vi "数据编码.vi"(0 "table输入":string(combo), 1 "仪器参数上传时间":enum16{"精确到小时", "原始时间"}(ring), 5 "错误常量 2":errorcluster caption="错误输入", 7 "仪器参数":string[](array[string]), 9 "QN":string, 11 "参数":string, 13 "MN":string, 14 "PW":string) -> (4 "错误常量":errorcluster caption="错误输出", 15 "通讯包字符串":string)   [LabVIEW 2016, in "数据传输系统-02.lvlib"]
panel:
  out "核查数据发送次数":i32
  out "小时数据发送次数":i32
  out "长度":i32
  in  "数据块":T1
  out "通讯包":T2={"包头（2）"="##", "数据段长度（4）"="", "数据段"="", "CRC校验"="", "包尾"=""}
  # "范例代码：\n\n##0101QN=20160801085857223;ST=32;CN=1062;PW=100000;MN=010000A8900016F000169DC0;Flag=5\n;CP=&&RtdInterval=30&&1C80\\r\\n"
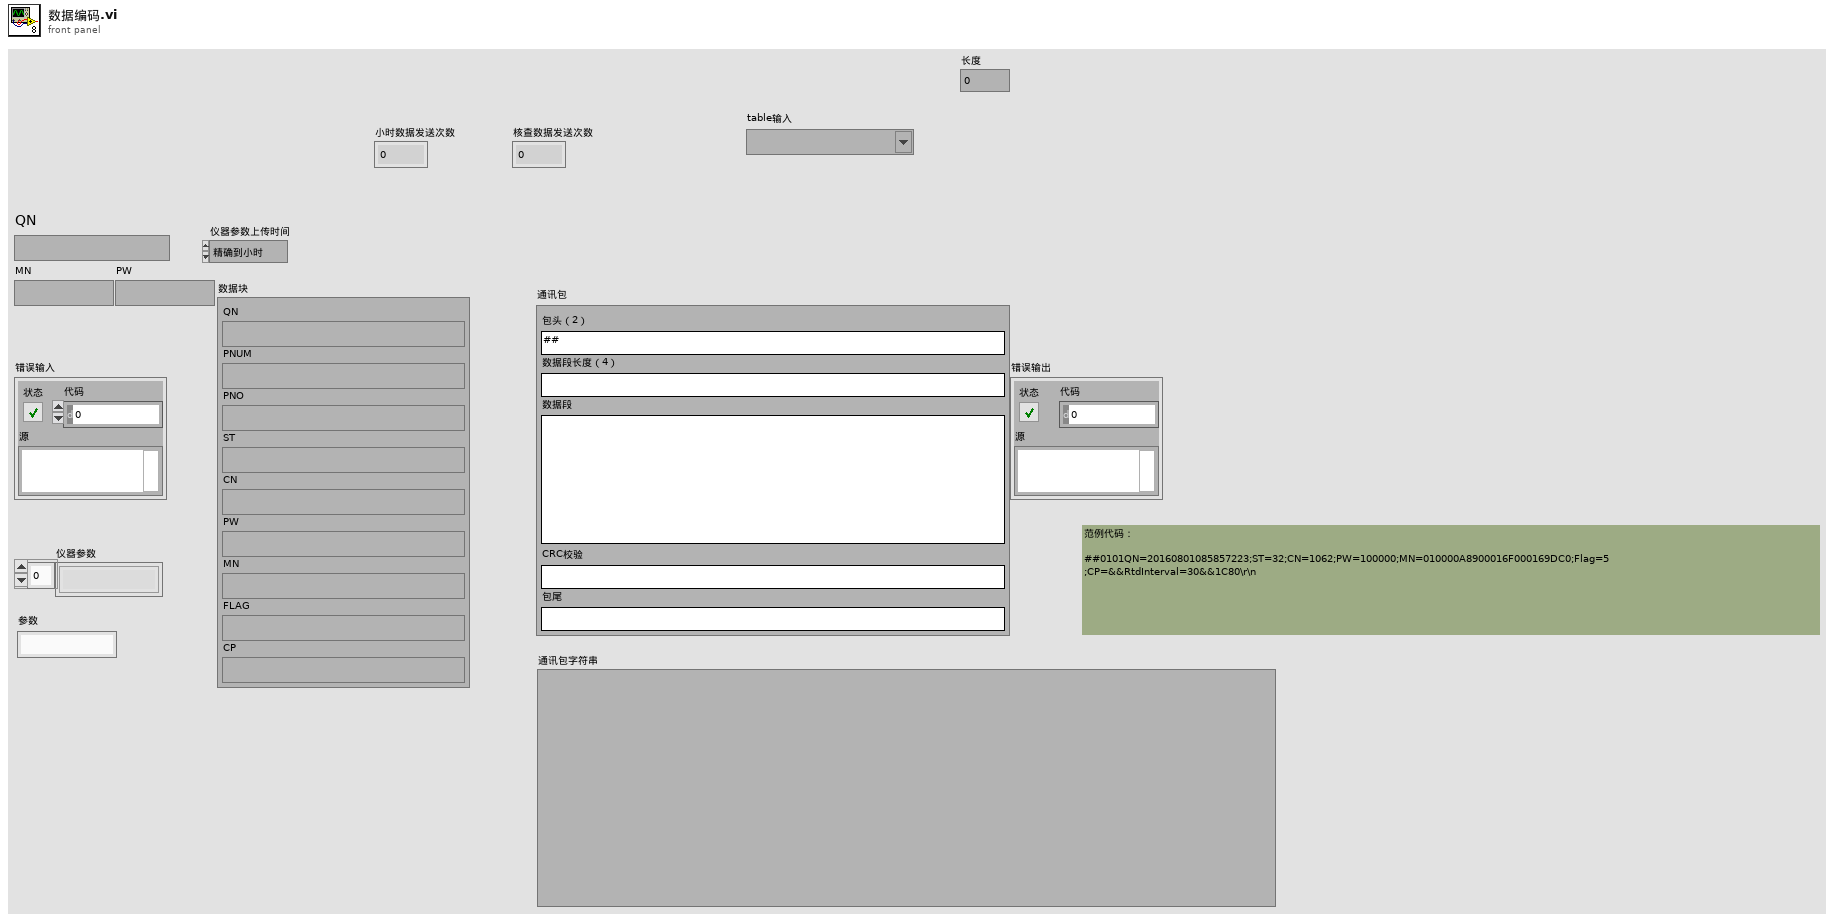
[diagram p1: front panel]
types:
  T1 = cluster{"QN":string, "ST":string, "CN":string, "PW":string, "MN":string, "FLAG":string, "PNUM":string, "PNO":string, "CP":string}
  T2 = cluster{"包头（2）":string, "数据段长度（4）":string, "数据段":string, "CRC校验":string, "包尾":string}
  T3 = cluster{"PH":string[][], "CODCr":string[][], "氨氮":string[][], "CODMn":string[][], "总氮":string[][], "总磷":string[][], "电导率":string[][], "水温":string[][], "DO":string[][], "浊度":string[][], "叶绿素":string[][], "藻密度":string[][], "铜":string[][], "盐度":string[][], "水位":string[][], "流速":string[][], "瞬时流量":string[][], "累积流量":string[][], "亚硝酸盐":string[][], "硫化物":string[][], "ORP":string[][], "铅":string[][], "镉":string[][], "锌":string[][], "镍":string[][], "锰":string[][], "汞":string[][], "气温":string[][], "气压":string[][], "风速":string[][], "风向":string[][], "盐度 2":string[][], "磷酸盐":string[][], "硝氮":string[][], "氟化物":string[][], "挥发酚":string[][], "氯化物":string[][]}
  T4 = enum16{"小时数据", "实时数据", "平行样测试", "集成干预测试", "加标回收测试", "核查数据", "空白零点跨度数据", "提取小时数据", "提取实时数据"}
  T5 = enum16{"小时数据", "实时数据", "平行样测试", "集成干预测试", "加标回收测试", "核查数据", "空白零点跨度数据", "提取小时数据", "提取实时数据", "操作日志"}
  T6 = enum16{"小时数据", "实时数据", "平行样测试", "集成干预测试", "加标回收测试", "核查数据", "空白零点跨度数据", "提取小时数据", "提取实时数据", "操作日志", "仪器参数", "3090仪器参数", "提取仪器参数", "报警信息"}
  T7 = cluster{"CODMn固件信息":string, "氨氮固件信息":string, "总磷固件信息":string, "总氮固件信息":string, "CODCr固件信息":string}
  T8 = typedef "数据传输系统-02.lvlib/应用环境.ctl" = enum16{"STD", "GB212", "婉仪平台"}
  T9 = cluster{"CODMn":dbl, "CODCr":dbl, "DO":dbl, "铜":dbl, "PH":dbl, "氨氮":dbl, "比电导率":dbl, "水温":dbl, "COD":dbl, "浊度":dbl, "总氮":dbl, "总磷":dbl, "叶绿素a":dbl, "藻密度":dbl, "水位":dbl, "流速":dbl, "瞬时流量":dbl, "累积流量":dbl, "亚硝酸盐":dbl, "硫化物":dbl, "ORP":dbl, "铅":dbl, "镉":dbl, "锌":dbl, "镍":dbl, "锰":dbl, "汞":dbl, "气温":dbl, "气压":dbl, "风速":dbl, "风向":dbl, "盐度":dbl, "磷酸盐":dbl, "硝氮":dbl, "氟化物":dbl, "挥发酚":dbl, "氯化物":dbl}
  T10 = cluster{"CODMn":string, "CODCr":string, "DO":string, "铜":string, "PH":string, "氨氮":string, "比电导率":string, "水温":string, "COD":string, "浊度":string, "总氮":string, "总磷":string, "叶绿素a":string, "藻密度":string, "水位":string, "流速":string, "瞬时流量":string, "累积流量":string, "亚硝酸盐":string, "硫化物":string, "ORP":string, "铅":string, "镉":string, "锌":string, "镍":string, "锰":string, "汞":string, "气温":string, "气压":string, "风速":string, "风向":string, "盐度":string, "磷酸盐":string, "硝氮":string, "氟化物":string, "挥发酚":string, "氯化物":string}
  T11 = typedef "LVDateTimeRec.ctl" = cluster{"秒数的小数部分":dbl, "秒":i32, "分":i32, "时":i32, "日":i32, "月":i32, "年":i32, "天数（周）":i32, "天数（年）":i32, "DST":i32}
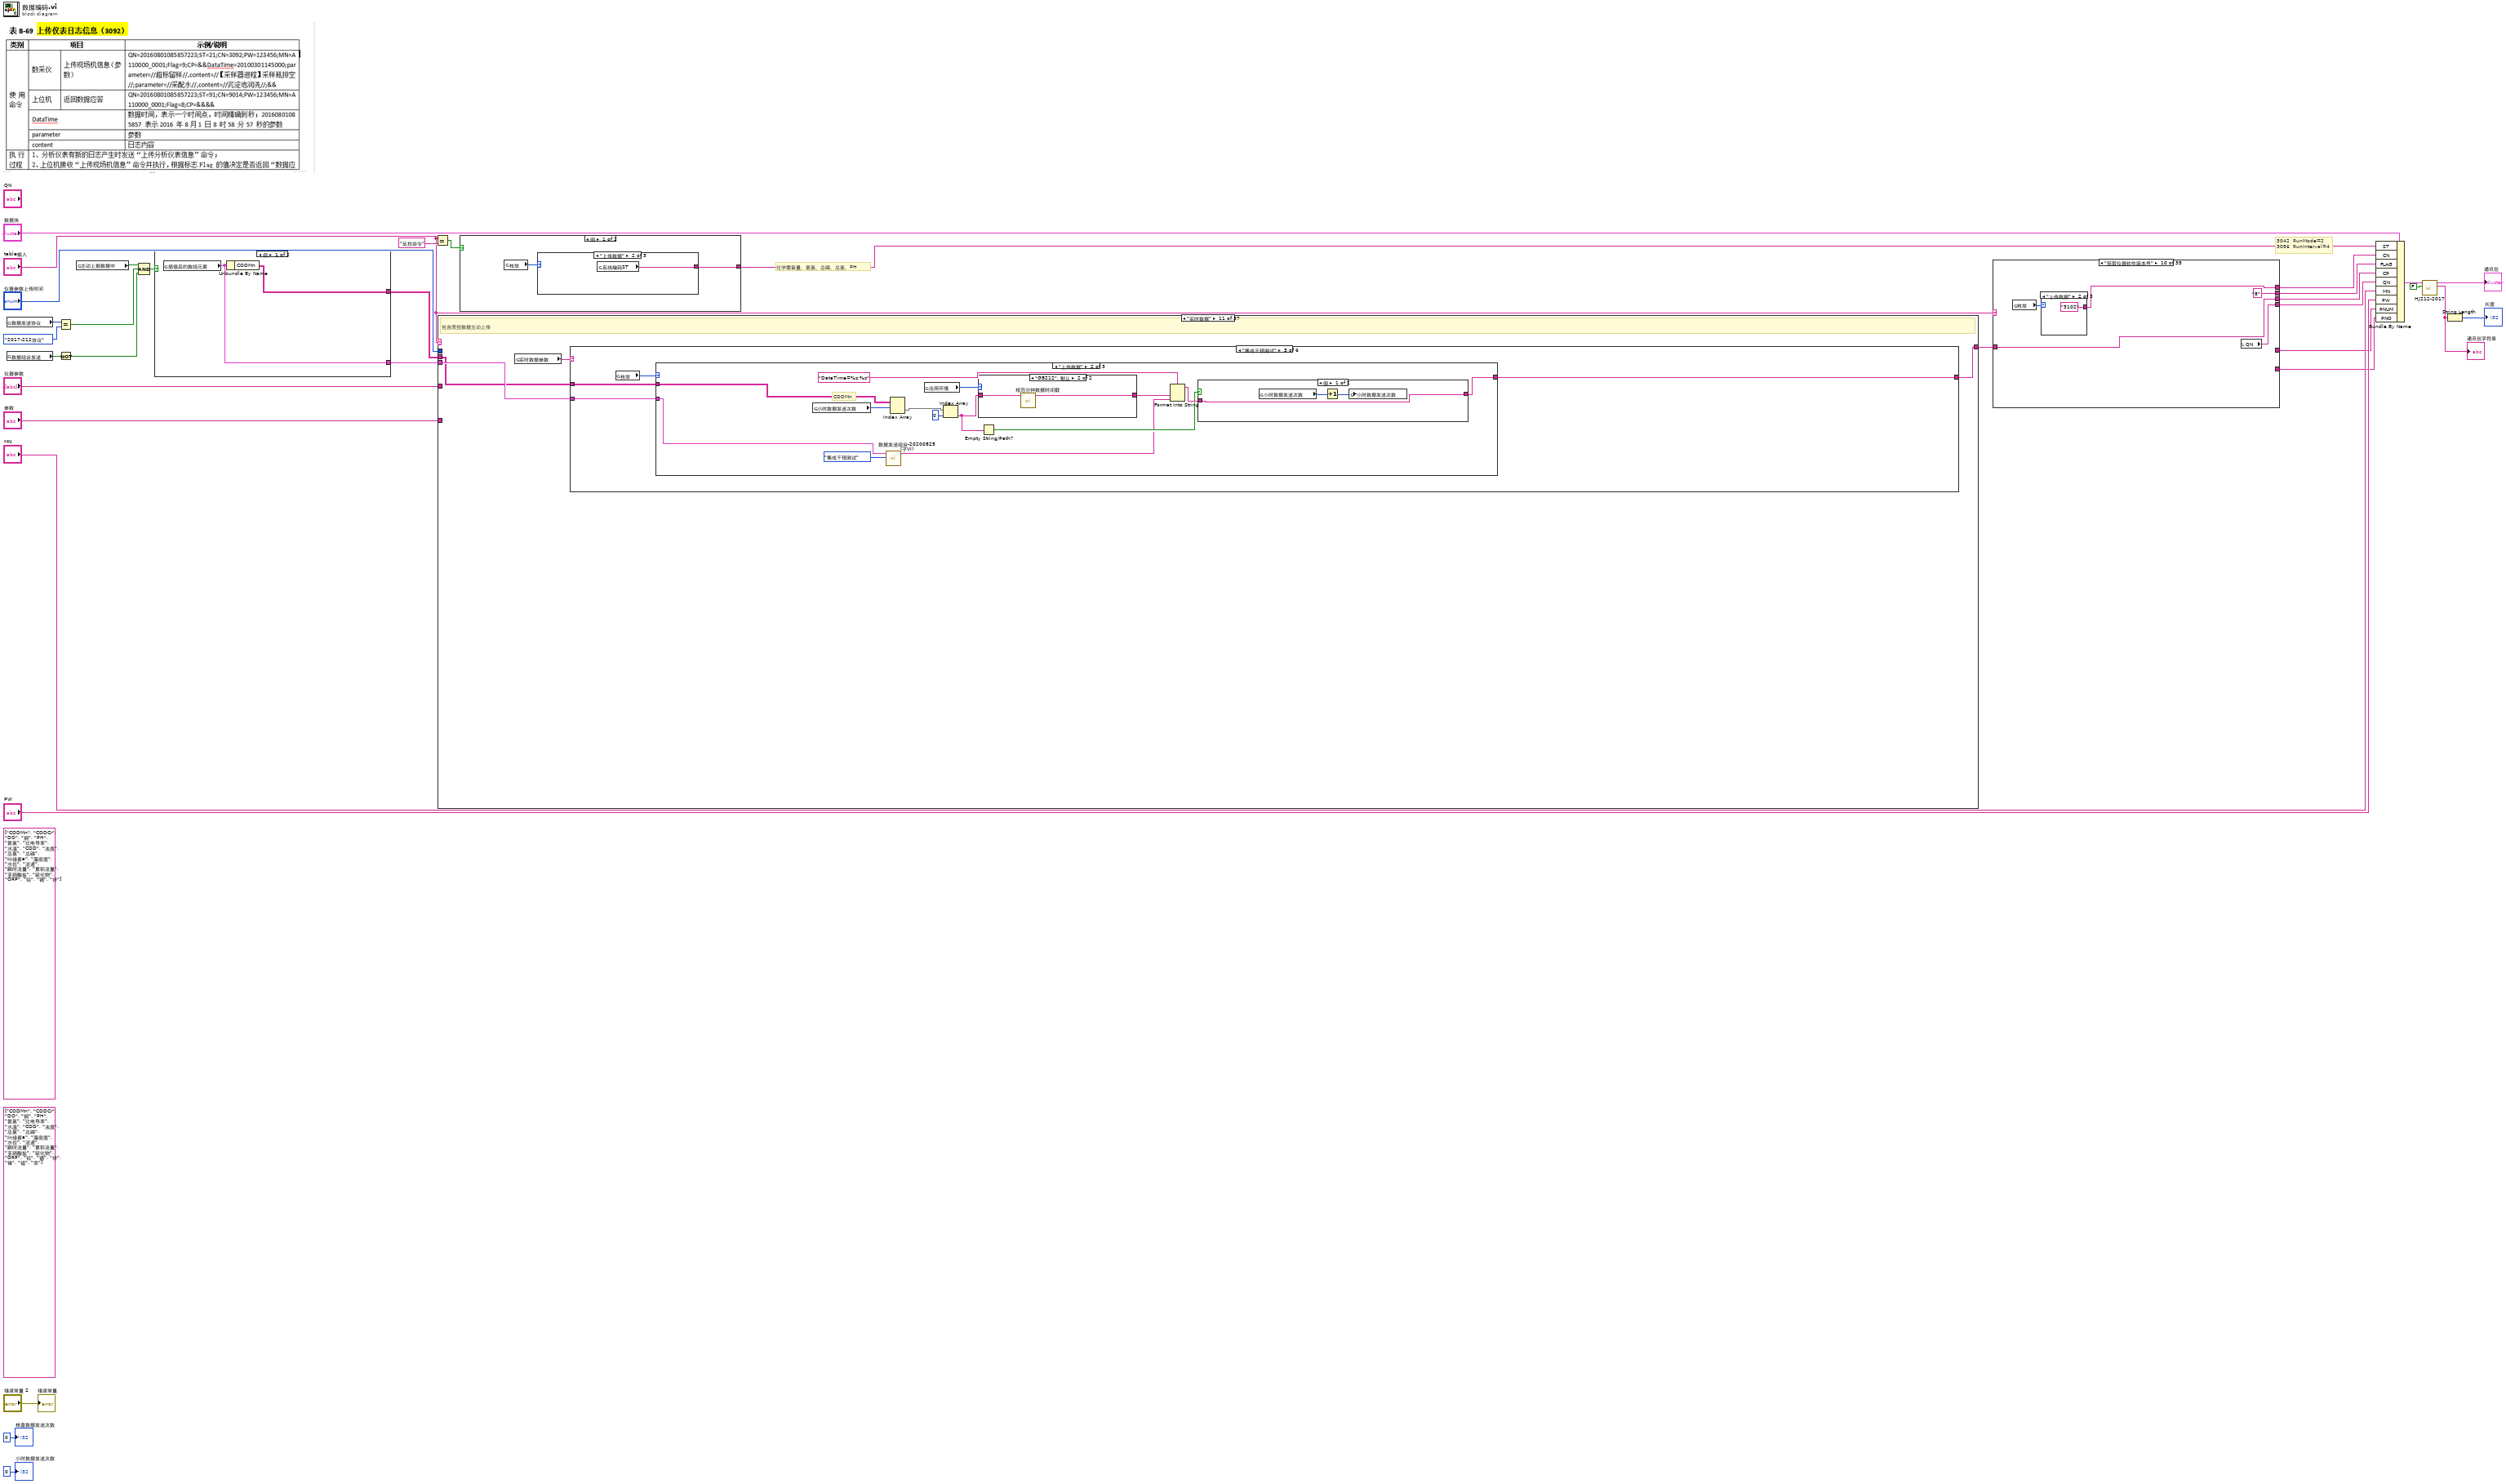
[diagram p0: block diagram]
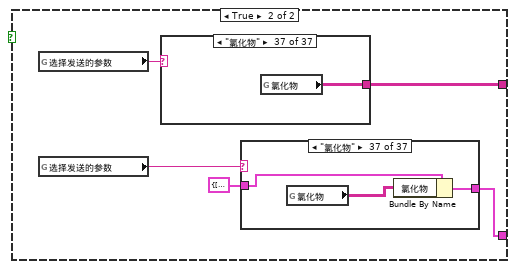
[diagram p2: hidden frame]
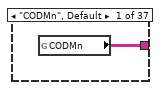
[diagram p3: hidden frame]
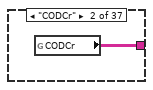
[diagram p4: hidden frame]
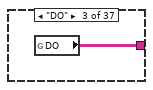
[diagram p5: hidden frame]
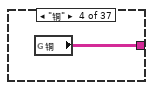
[diagram p6: hidden frame]
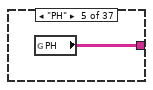
[diagram p7: hidden frame]
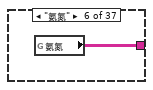
[diagram p8: hidden frame]
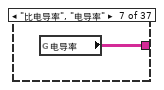
[diagram p9: hidden frame]
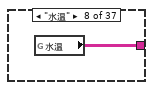
[diagram p10: hidden frame]
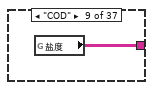
[diagram p11: hidden frame]
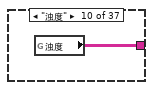
[diagram p12: hidden frame]
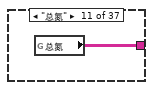
[diagram p13: hidden frame]
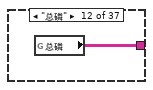
[diagram p14: hidden frame]
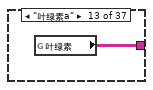
[diagram p15: hidden frame]
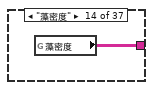
[diagram p16: hidden frame]
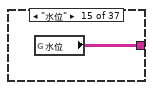
[diagram p17: hidden frame]
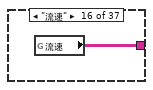
[diagram p18: hidden frame]
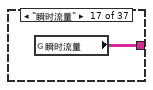
[diagram p19: hidden frame]
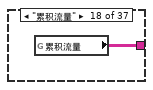
[diagram p20: hidden frame]
diagram:
  (unwired) string[] ["CODMn", "CODCr", "DO", "铜", "PH", "氨氮", "比电导率", "水温", "COD", "浊度", "总氮", "总磷", "叶绿素a", "藻密度", "水位", "流速", "瞬时流量", "累积流量", "亚硝酸盐", "硫化物", "ORP", "铅", "镉", "锌"] ("数组")
  (unwired) string[] ["CODMn", "CODCr", "DO", "铜", "PH", "氨氮", "比电导率", "水温", "COD", "浊度", "总氮", "总磷", "叶绿素a", "藻密度", "水位", "流速", "瞬时流量", "累积流量", "亚硝酸盐", "硫化物", "ORP", "铅", "镉", "锌", "镍", "锰", "汞"] ("数组")
  # "化学需氧量、氨氮、总磷、总氮、PH"
  # "3042  RunMode=2\n3056  RunInterval=4"
  n1 = global read "断电保存全局.vi" "数据发送协议"() -> (w11:enum16{"2005-212协议", "2017-212协议"})
  n2 = global read "断电保存全局.vi" "数据组合发送"() -> (w13:bool)
  n3 = Equal?(x=w11, y=enum16{"2005-212协议", "2017-212协议"}."2017-212协议" ("数据发送版本")) -> (x = y?=w14:bool)
  n4 = Not(x=w13) -> (.not. x?=w12:bool)
  n5 = global read "全局 数据发送重叠.vi" "主动上报数据中"() -> (w18:bool)
  n6 = Compound Arithmetic op=AND ("复合运算")(w18, w14, w12) -> (w15:bool)
  n7 = case shown="假" w15 {
    tunnel: [w36 w40] -> w9
    tunnel: [w35 w38] -> w7
    frame False {
      n8 = global read "插值后的新数组.vi" "插值后的数组元素"() -> (w36:T3)
      n9 = Unbundle By Name(w36) -> ("CODMn"=w35:string[][])
    }
    frame True {
      n10 = global read "全局 水样时间.vi" "选择发送的参数"() -> (w39:string)
      n11 = global read "全局 水样时间.vi" "选择发送的参数"() -> (w41:string)
      n12 = case shown="\"氯化物\"" w39 {
        tunnel: [w42 w43 w44 w45 w46 w47 w48 w49 w50 w51 w52 w53 w54 w55 w56 w57 w58 w59 w60 w61 w62 w63 w64 w65 w66 w67 w68 w69 w70 w71 w72 w73 w74 w75 w76 w77 w78] -> w38
        frame "CODMn", Default {
          n13 = global read "全局 所有参数.vi" "CODMn"() -> (w42:string[][])
        }
        frame "CODCr" {
          n14 = global read "全局 所有参数.vi" "CODCr"() -> (w43:string[][])
        }
        frame "DO" {
          n15 = global read "全局 所有参数.vi" "DO"() -> (w44:string[][])
        }
        frame "铜" {
          n16 = global read "全局 所有参数.vi" "铜"() -> (w45:string[][])
        }
        frame "PH" {
          n17 = global read "全局 所有参数.vi" "PH"() -> (w46:string[][])
        }
        frame "氨氮" {
          n18 = global read "全局 所有参数.vi" "氨氮"() -> (w47:string[][])
        }
        frame "比电导率", "电导率" {
          n19 = global read "全局 所有参数.vi" "电导率"() -> (w48:string[][])
        }
        frame "水温" {
          n20 = global read "全局 所有参数.vi" "水温"() -> (w49:string[][])
        }
        frame "COD" {
          n21 = global read "全局 所有参数.vi" "盐度"() -> (w50:string[][])
        }
        frame "浊度" {
          n22 = global read "全局 所有参数.vi" "浊度"() -> (w51:string[][])
        }
        frame "总氮" {
          n23 = global read "全局 所有参数.vi" "总氮"() -> (w52:string[][])
        }
        frame "总磷" {
          n24 = global read "全局 所有参数.vi" "总磷"() -> (w53:string[][])
        }
        frame "叶绿素a" {
          n25 = global read "全局 所有参数.vi" "叶绿素"() -> (w54:string[][])
        }
        frame "藻密度" {
          n26 = global read "全局 所有参数.vi" "藻密度"() -> (w55:string[][])
        }
        frame "水位" {
          n27 = global read "全局 所有参数.vi" "水位"() -> (w56:string[][])
        }
        frame "流速" {
          n28 = global read "全局 所有参数.vi" "流速"() -> (w57:string[][])
        }
        frame "瞬时流量" {
          n29 = global read "全局 所有参数.vi" "瞬时流量"() -> (w58:string[][])
        }
        frame "累积流量" {
          n30 = global read "全局 所有参数.vi" "累积流量"() -> (w59:string[][])
        }
        frame "亚硝氮" {
          n31 = global read "全局 所有参数.vi" "亚硝酸盐"() -> (w60:string[][])
        }
        frame "硫化物" {
          n32 = global read "全局 所有参数.vi" "硫化物"() -> (w61:string[][])
        }
        frame "ORP" {
          n33 = global read "全局 所有参数.vi" "ORP"() -> (w62:string[][])
        }
        frame "铅" {
          n34 = global read "全局 所有参数.vi" "铅"() -> (w63:string[][])
        }
        frame "镉" {
          n35 = global read "全局 所有参数.vi" "镉"() -> (w64:string[][])
        }
        frame "锌" {
          n36 = global read "全局 所有参数.vi" "锌"() -> (w65:string[][])
        }
        frame "镍" {
          n37 = global read "全局 所有参数.vi" "镍"() -> (w66:string[][])
        }
        frame "锰" {
          n38 = global read "全局 所有参数.vi" "锰"() -> (w67:string[][])
        }
        frame "汞" {
          n39 = global read "全局 所有参数.vi" "汞"() -> (w68:string[][])
        }
        frame "气温" {
          n40 = global read "全局 所有参数.vi" "气温"() -> (w69:string[][])
        }
        frame "气压" {
          n41 = global read "全局 所有参数.vi" "气压"() -> (w70:string[][])
        }
        frame "风速" {
          n42 = global read "全局 所有参数.vi" "风速"() -> (w71:string[][])
        }
        frame "风向" {
          n43 = global read "全局 所有参数.vi" "风向"() -> (w72:string[][])
        }
        frame "盐度" {
          n44 = global read "全局 所有参数.vi" "盐度 2"() -> (w73:string[][])
        }
        frame "磷酸盐" {
          n45 = global read "全局 所有参数.vi" "磷酸盐"() -> (w74:string[][])
        }
        frame "硝氮" {
          n46 = global read "全局 所有参数.vi" "硝氮"() -> (w75:string[][])
        }
        frame "氟化物" {
          n47 = global read "全局 所有参数.vi" "氟化物"() -> (w76:string[][])
        }
        frame "挥发酚" {
          n48 = global read "全局 所有参数.vi" "挥发酚"() -> (w77:string[][])
        }
        frame "氯化物" {
          n49 = global read "全局 所有参数.vi" "氯化物"() -> (w78:string[][])
        }
      }
      n50 = case shown="\"氯化物\"" w41 {
        tunnel: T3 {"PH"=[], "CODCr"=[], "氨氮"=[], "CODMn"=[], "总氮"=[], "总磷"=[], "电导率"=[], "水温"=[], "DO"=[], "浊度"=[], "叶绿素"=[], "藻密度"=[], "铜"=[], "盐度"=[], "水位"=[], "流速"=[], "瞬时流量"=[], "累积流量"=[], "亚硝酸盐"=[], "硫化物"=[], "ORP"=[], "铅"=[], "镉"=[], "锌"=[], "镍"=[], "锰"=[], "汞"=[], "气温"=[], "气压"=[], "风速"=[], "风向"=[], "盐度 2"=[], "磷酸盐"=[], "硝氮"=[], "氟化物"=[], "挥发酚"=[], "氯化物"=[]} ("插值后的数组元素") -> [w80 w84 w87 w90 w93 w96 w99 w102 w105 w108 w111 w114 w117 w119 w123 w126 w128 w131 w134 w137 w140 w143 w146 w149 w152 w155 w158 w161 w164 w167 w170 w173 w176 w179 w182 w185 w188]
        tunnel: [w79 w82 w85 w88 w91 w94 w98 w101 w103 w106 w109 w112 w115 w118 w121 w124 w127 w130 w133 w136 w139 w142 w145 w148 w151 w154 w157 w160 w163 w166 w169 w172 w175 w178 w181 w184 w187] -> w40
        frame "CODMn", Default {
          n51 = global read "全局 所有参数.vi" "CODMn"() -> (w81:string[][])
          n52 = Bundle By Name(cluster=w80, "CODMn"=w81) -> (w79:T3)
        }
        frame "CODCr" {
          n53 = global read "全局 所有参数.vi" "CODCr"() -> (w83:string[][])
          n54 = Bundle By Name(cluster=w84, "CODCr"=w83) -> (w82:T3)
        }
        frame "DO" {
          n55 = global read "全局 所有参数.vi" "DO"() -> (w86:string[][])
          n56 = Bundle By Name(cluster=w87, "DO"=w86) -> (w85:T3)
        }
        frame "铜" {
          n57 = global read "全局 所有参数.vi" "铜"() -> (w89:string[][])
          n58 = Bundle By Name(cluster=w90, "铜"=w89) -> (w88:T3)
        }
        frame "PH" {
          n59 = global read "全局 所有参数.vi" "PH"() -> (w92:string[][])
          n60 = Bundle By Name(cluster=w93, "PH"=w92) -> (w91:T3)
        }
        frame "氨氮" {
          n61 = global read "全局 所有参数.vi" "氨氮"() -> (w95:string[][])
          n62 = Bundle By Name(cluster=w96, "氨氮"=w95) -> (w94:T3)
        }
        frame "比电导率", "电导率" {
          n63 = global read "全局 所有参数.vi" "电导率"() -> (w97:string[][])
          n64 = Bundle By Name(cluster=w99, "电导率"=w97) -> (w98:T3)
        }
        frame "水温" {
          n65 = global read "全局 所有参数.vi" "水温"() -> (w100:string[][])
          n66 = Bundle By Name(cluster=w102, "水温"=w100) -> (w101:T3)
        }
        frame "COD" {
          n67 = global read "全局 所有参数.vi" "盐度"() -> (w104:string[][])
          n68 = Bundle By Name(cluster=w105, "盐度"=w104) -> (w103:T3)
        }
        frame "浊度" {
          n69 = global read "全局 所有参数.vi" "浊度"() -> (w107:string[][])
          n70 = Bundle By Name(cluster=w108, "浊度"=w107) -> (w106:T3)
        }
        frame "总氮" {
          n71 = global read "全局 所有参数.vi" "总氮"() -> (w110:string[][])
          n72 = Bundle By Name(cluster=w111, "总氮"=w110) -> (w109:T3)
        }
        frame "总磷" {
          n73 = global read "全局 所有参数.vi" "总磷"() -> (w113:string[][])
          n74 = Bundle By Name(cluster=w114, "总磷"=w113) -> (w112:T3)
        }
        frame "叶绿素a" {
          n75 = global read "全局 所有参数.vi" "叶绿素"() -> (w116:string[][])
          n76 = Bundle By Name(cluster=w117, "叶绿素"=w116) -> (w115:T3)
        }
        frame "藻密度" {
          n77 = global read "全局 所有参数.vi" "藻密度"() -> (w120:string[][])
          n78 = Bundle By Name(cluster=w119, "藻密度"=w120) -> (w118:T3)
        }
        frame "水位" {
          n79 = global read "全局 所有参数.vi" "水位"() -> (w122:string[][])
          n80 = Bundle By Name(cluster=w123, "水位"=w122) -> (w121:T3)
        }
        frame "流速" {
          n81 = global read "全局 所有参数.vi" "流速"() -> (w125:string[][])
          n82 = Bundle By Name(cluster=w126, "流速"=w125) -> (w124:T3)
        }
        frame "瞬时流量" {
          n83 = global read "全局 所有参数.vi" "瞬时流量"() -> (w129:string[][])
          n84 = Bundle By Name(cluster=w128, "瞬时流量"=w129) -> (w127:T3)
        }
        frame "累积流量" {
          n85 = global read "全局 所有参数.vi" "累积流量"() -> (w132:string[][])
          n86 = Bundle By Name(cluster=w131, "累积流量"=w132) -> (w130:T3)
        }
        frame "亚硝氮" {
          n87 = global read "全局 所有参数.vi" "亚硝酸盐"() -> (w135:string[][])
          n88 = Bundle By Name(cluster=w134, "亚硝酸盐"=w135) -> (w133:T3)
        }
        frame "硫化物" {
          n89 = global read "全局 所有参数.vi" "硫化物"() -> (w138:string[][])
          n90 = Bundle By Name(cluster=w137, "硫化物"=w138) -> (w136:T3)
        }
        frame "ORP" {
          n91 = global read "全局 所有参数.vi" "ORP"() -> (w141:string[][])
          n92 = Bundle By Name(cluster=w140, "ORP"=w141) -> (w139:T3)
        }
        frame "铅" {
          n93 = global read "全局 所有参数.vi" "铅"() -> (w144:string[][])
          n94 = Bundle By Name(cluster=w143, "铅"=w144) -> (w142:T3)
        }
        frame "镉" {
          n95 = global read "全局 所有参数.vi" "镉"() -> (w147:string[][])
          n96 = Bundle By Name(cluster=w146, "镉"=w147) -> (w145:T3)
        }
        frame "锌" {
          n97 = global read "全局 所有参数.vi" "锌"() -> (w150:string[][])
          n98 = Bundle By Name(cluster=w149, "锌"=w150) -> (w148:T3)
        }
        frame "镍" {
          n99 = global read "全局 所有参数.vi" "镍"() -> (w153:string[][])
          n100 = Bundle By Name(cluster=w152, "镍"=w153) -> (w151:T3)
        }
        frame "锰" {
          n101 = global read "全局 所有参数.vi" "锰"() -> (w156:string[][])
          n102 = Bundle By Name(cluster=w155, "锰"=w156) -> (w154:T3)
        }
        frame "汞" {
          n103 = global read "全局 所有参数.vi" "汞"() -> (w159:string[][])
          n104 = Bundle By Name(cluster=w158, "汞"=w159) -> (w157:T3)
        }
        frame "气温" {
          n105 = global read "全局 所有参数.vi" "气温"() -> (w162:string[][])
          n106 = Bundle By Name(cluster=w161, "气温"=w162) -> (w160:T3)
        }
        frame "气压" {
          n107 = global read "全局 所有参数.vi" "气压"() -> (w165:string[][])
          n108 = Bundle By Name(cluster=w164, "气压"=w165) -> (w163:T3)
        }
        frame "风速" {
          n109 = global read "全局 所有参数.vi" "风速"() -> (w168:string[][])
          n110 = Bundle By Name(cluster=w167, "风速"=w168) -> (w166:T3)
        }
        frame "风向" {
          n111 = global read "全局 所有参数.vi" "风向"() -> (w171:string[][])
          n112 = Bundle By Name(cluster=w170, "风向"=w171) -> (w169:T3)
        }
        frame "盐度" {
          n113 = global read "全局 所有参数.vi" "盐度 2"() -> (w174:string[][])
          n114 = Bundle By Name(cluster=w173, "盐度 2"=w174) -> (w172:T3)
        }
        frame "磷酸盐" {
          n115 = global read "全局 所有参数.vi" "磷酸盐"() -> (w177:string[][])
          n116 = Bundle By Name(cluster=w176, "磷酸盐"=w177) -> (w175:T3)
        }
        frame "硝氮" {
          n117 = global read "全局 所有参数.vi" "硝氮"() -> (w180:string[][])
          n118 = Bundle By Name(cluster=w179, "硝氮"=w180) -> (w178:T3)
        }
        frame "氟化物" {
          n119 = global read "全局 所有参数.vi" "氟化物"() -> (w183:string[][])
          n120 = Bundle By Name(cluster=w182, "氟化物"=w183) -> (w181:T3)
        }
        frame "挥发酚" {
          n121 = global read "全局 所有参数.vi" "挥发酚"() -> (w186:string[][])
          n122 = Bundle By Name(cluster=w185, "挥发酚"=w186) -> (w184:T3)
        }
        frame "氯化物" {
          n123 = global read "全局 所有参数.vi" "氯化物"() -> (w189:string[][])
          n124 = Bundle By Name(cluster=w188, "氯化物"=w189) -> (w187:T3)
        }
      }
    }
  }
  n125 = Equal?(x="table输入", y="反控命令") -> (x = y?=w24:bool)
  n126 = case shown="\"实时数据\"" "table输入" {
    tunnel: [w191 w198 w212 w254 w292 _ w306 w315 w322 w332 w343 w498 w529 w580 w628 w680 w709 w741 w772 w798 w827 w856 w893 w926 w959 w998 w1159 w1201 w1362 w1390 w1413 w1446 w1469 w1480 w1488 w1498 w1508] -> w19
    tunnel: w7 -> [_ _ _ _ _ _ _ _ _ _ w340 w497 _ _ _ w679 w710 w736 w767 w799 w826 w855 w892 _ _ _ _ _ w1361 _ w1412 _ _ _ _ _ _]
    tunnel: w9 -> [_ _ _ _ _ _ _ _ _ _ w341 w499 _ _ _ w675 w705 w737 w768 w797 w825 w854 w888 _ _ _ _ _ w1357 w1388 w1408 _ _ _ _ _ _]
    tunnel: "仪器参数" -> [_ _ _ _ _ _ _ _ _ _ _ _ _ _ _ _ _ _ _ _ _ _ _ _ _ w994 w1157 w1197 _ _ _ _ _ _ _ _ _]
    tunnel: "参数" -> [_ _ _ _ _ _ _ _ _ _ _ _ _ _ _ _ _ _ _ _ _ _ _ _ _ w996 _ w1199 _ _ _ _ _ _ _ _ _]
    tunnel: "仪器参数上传时间" -> [_ _ _ _ _ _ _ _ _ _ _ _ _ _ _ _ _ _ _ _ _ _ _ _ _ w993 w1156 w1196 _ _ _ _ _ _ _ _ _]
    frame "反控命令" {
      n127 = global read "全局 反控命令枚举.vi" "反控命令枚举"() -> (w190:enum16{"返回请求应答", "返回执行结果"})
      n128 = case shown="\"返回执行结果\"" w190 {
        tunnel: ["QnRtn=1" w194] -> w191
        frame "返回请求应答", Default {
        }
        frame "返回执行结果" {
          n129 = global read "全局 反控命令枚举.vi" "执行结果定义"() -> (w195:u16)
          n130 = Number To Decimal String(number=w195) -> (decimal integer string=w193:string)  [unwired: 1 in]
          n131 = Concatenate Strings("ExeRtn=", w193) -> (w194:string)
        }
      }
    }
    frame "超标留样返回" {
      n132 = global read "全局1.vi" "枚举"() -> (w197:enum16{"返回请求应答", "上传数据", "返回执行结果"})
      n133 = case shown="\"返回执行结果\"" w197 {
        tunnel: ["QnRtn=1" w200 "ExeRtn=1"] -> w198
        frame "返回请求应答", Default {
        }
        frame "上传数据" {
          n134 = global read "全局1.vi" "register values"() -> (w209:u16[])
          n135 = Get Date/Time In Seconds() -> (seconds since 1Jan1904=w207:timestamp)
          n136 = Index Array(array=w209, index=7 ("索引")) -> (element=w202:u16)
          n137 = Format Date/Time String(time format string (%c)="%Y%m%d%H%M%S" ("时间格式字符串(%c)"), seconds (now)=w207) -> (date/time string=w205:string)  [unwired: 1 in]
          n138 = Number To Decimal String(number=w202) -> (decimal integer string=w203:string)  [unwired: 1 in]
          n139 = Format Into String(format string="VaseNo=%s" ("格式字符串"), w203) -> (resulting string=w201:string)  [unwired: 2 in, 1 out]
          n140 = Format Into String(format string="DataTime=%s;%s" ("格式字符串"), w205, w201) -> (resulting string=w200:string)  [unwired: 2 in, 1 out]
        }
        frame "返回执行结果" {
        }
      }
    }
    frame "提取经纬度环境信息" {
      # "BDS纬度"
      # "BDS纬度"
      # "GPS纬度"
      # "GPS经度"
      # "湿度"
      # "温度"
      # "电压"
      # "时间"
      n141 = global read "全局1.vi" "枚举"() -> (w213:enum16{"返回请求应答", "上传数据", "返回执行结果"})
      n142 = case shown="\"上传数据\"" w213 {
        tunnel: ["QnRtn=1" w226 "ExeRtn=1"] -> w212
        frame "返回请求应答", Default {
        }
        frame "上传数据" {
          n143 = global read "全局 环境参数.vi" "环境参数"() -> (w216:string[][])
          n144 = global read "全局 环境参数.vi" "columns输出"() -> (w223:string[])
          n145 = Index Array(array=w216, index (row)=0 ("索引 (行)")) -> (element=w219:string[])  [unwired: 1 in]
          n146 = Get Date/Time In Seconds() -> (seconds since 1Jan1904=w228:timestamp)
          n147 = Array Subset(array=w223, index=1 ("索引")) -> (w224:string[])  [unwired: 1 in]
          n148 = for {
            tunnel: w224 -> [w232] mode=indexing
            tunnel: [w231] -> w225 mode=indexing
            n149 = case shown="\"BDS经度\"" w232 {
              tunnel: ["" "Volt=%s;" "Temp=%s;" ("格式字符串") "Hum=%s;" ("格式字符串") "Lng=%s;" "Lat=%s;" "Lng2=%s;" "Lat2=%s;"] -> w231
              frame "假", Default {
              }
              frame "电压" {
              }
              frame "室温" {
              }
              frame "湿度" {
              }
              frame "GPS经度" {
              }
              frame "GPS纬度" {
              }
              frame "BDS经度" {
              }
              frame "BDS纬度" {
              }
            }
          }
          n150 = Format Date/Time String(time format string (%c)="%Y%m%d%H%M%S" ("时间格式字符串(%c)"), seconds (now)=w228) -> (date/time string=w227:string)  [unwired: 1 in]
          n151 = Array Subset(array=w219, index=1 ("索引")) -> (w221:string[])  [unwired: 1 in]
          n152 = for {
            shift-right: [w246] -> w215
            shift-left: "" -> [w245]
            tunnel: w225 -> [w244] mode=indexing
            tunnel: w221 -> [w242] mode=indexing
            n153 = Empty String/Path?(string/path=w242) -> (empty?=w248:bool)
            n154 = Fract/Exp String To Number(string=w242) -> (number=w243:dbl)  [unwired: 3 in, 1 out]
            n155 = Number To Fractional String(number=w243) -> (F-format string=w241:string)  [unwired: 3 in]
            n156 = case shown="假" w248 {
              tunnel: [w251 w252] -> w247
              tunnel: w244 -> [w250 _]
              tunnel: w241 -> [w249 _]
              tunnel: w241 -> [_ w252]
              frame False {
                n157 = Format Into String(format string=w250, w249) -> (resulting string=w251:string)  [unwired: 2 in, 1 out]
              }
              frame True {
              }
            }
            n158 = Concatenate Strings(w245, w247) -> (w246:string)
          }
          n159 = Format Into String(format string="DataTime=%s;%s" ("格式字符串"), w227, w215) -> (resulting string=w226:string)  [unwired: 2 in, 1 out]
        }
        frame "返回执行结果" {
        }
      }
    }
    frame "提取现场系统信息" {
      n160 = global read "全局1.vi" "枚举"() -> (w255:enum16{"返回请求应答", "上传数据", "返回执行结果"})
      n161 = case shown="\"上传数据\"" w255 {
        tunnel: ["QnRtn=1" w289 "ExeRtn=1"] -> w254
        frame "返回请求应答", Default {
        }
        frame "上传数据" {
          n162 = global read "全局1.vi" "register values"() -> (w288:u16[])
          n163 = global read "全局1.vi" "系统信息"() -> (w270:u16[])
          n164 = Get Date/Time In Seconds() -> (seconds since 1Jan1904=w275:timestamp)
          n165 = Format Date/Time String(time format string (%c)="%Y%m%d%H%M%S%u" ("时间格式字符串(%c)"), seconds (now)=w275) -> (date/time string=w278:string)  [unwired: 1 in]
          n166 = Number To Decimal String(number=w270) -> (decimal integer string=w269:string[])  [unwired: 1 in]
          n167 = Index Array(array=w288, index #1=0 ("索引"), index #2=6 ("索引")) -> (element #1=w284:u16, element #2=w272:u16)
          n168 = Number To Decimal String(number=w284) -> (decimal integer string=w286:string)  [unwired: 1 in]
          n169 = Number To Decimal String(number=w272) -> (decimal integer string=w281:string)  [unwired: 1 in]
          n170 = Index Array(array=w269) -> (element #1=w267:string, element #2=w264:string, element #3=w261:string, element #4=w258:string)  [unwired: 4 in]
          n171 = Search and Replace String(input string=w278, search string="." ("搜索字符串")) -> (result string=w274:string)  [unwired: 6 in, 3 out]
          n172 = Format Into String(format string="SystemTask=%s;" ("格式字符串"), w267) -> (resulting string=w266:string)  [unwired: 2 in, 1 out]
          n173 = Format Into String(format string="PumpState=%s;" ("格式字符串"), w264) -> (resulting string=w263:string)  [unwired: 2 in, 1 out]
          n174 = Format Into String(format string="AlgClean=%s;" ("格式字符串"), w261) -> (resulting string=w260:string)  [unwired: 2 in, 1 out]
          n175 = Format Into String(format string="SystemAlarm=0%s;" ("格式字符串"), w258) -> (resulting string=w257:string)  [unwired: 2 in, 1 out]
          n176 = Format Into String(format string="RunMode=%s;" ("格式字符串"), w286) -> (resulting string=w271:string)  [unwired: 2 in, 1 out]
          n177 = Format Into String(format string="RunInterval=%s;" ("格式字符串"), w281) -> (resulting string=w282:string)  [unwired: 2 in, 1 out]
          n178 = Format Into String(format string="SystemTime=%s;" ("格式字符串"), w274) -> (resulting string=w279:string)  [unwired: 2 in, 1 out]
          n179 = Concatenate Strings(w271, w263, w266, w260, w257, w282, w279) -> (w289:string)
        }
        frame "返回执行结果" {
        }
      }
    }
    frame "提取监测仪表时间" {
      n180 = global read "全局1.vi" "枚举"() -> (w291:enum16{"返回请求应答", "上传数据", "返回执行结果"})
      n181 = case shown="\"上传数据\"" w291 {
        tunnel: ["QnRtn=1" w304 "ExeRtn=1"] -> w292
        frame "返回请求应答", Default {
        }
        frame "上传数据" {
          n182 = global read "全局 提取仪器参数.vi" "仪器编码"() -> (w294:string)
          n183 = Format Into String(format string="PolId=%s;" ("格式字符串"), w294) -> (resulting string=w302:string)  [unwired: 2 in, 1 out]
          n184 = Get Date/Time In Seconds() -> (seconds since 1Jan1904=w297:timestamp)
          n185 = Format Date/Time String(time format string (%c)="%Y%m%d%H%M%S%u" ("时间格式字符串(%c)"), seconds (now)=w297) -> (date/time string=w300:string)  [unwired: 1 in]
          n186 = Search and Replace String(input string=w300, search string="." ("搜索字符串")) -> (result string=w296:string)  [unwired: 6 in, 3 out]
          n187 = Format Into String(format string="SystemTime=%s;" ("格式字符串"), w296) -> (resulting string=w295:string)  [unwired: 2 in, 1 out]
          n188 = Concatenate Strings(w302, w295) -> (w304:string)
        }
        frame "返回执行结果" {
        }
      }
    }
    frame "心跳包", Default {
    }
    frame "提取数采仪时间" {
      (unwired) ""
      n189 = global read "全局1.vi" "枚举"() -> (w307:enum16{"返回请求应答", "上传数据", "返回执行结果"})
      n190 = case shown="\"上传数据\"" w307 {
        tunnel: ["QnRtn=1" w309 "ExeRtn=1"] -> w306
        frame "返回请求应答", Default {
        }
        frame "上传数据" {
          n191 = Get Date/Time In Seconds() -> (seconds since 1Jan1904=w313:timestamp)
          n192 = Format Date/Time String(time format string (%c)="%Y%m%d%H%M%S" ("时间格式字符串(%c)"), seconds (now)=w313) -> (date/time string=w310:string)  [unwired: 1 in]
          n193 = Concatenate Strings("SystemTime=", w310) -> (w309:string)
        }
        frame "返回执行结果" {
        }
      }
    }
    frame "获取软件版本号" {
      (unwired) ""
      n194 = global read "全局1.vi" "枚举"() -> (w316:enum16{"返回请求应答", "上传数据", "返回执行结果"})
      n195 = case shown="\"上传数据\"" w316 {
        tunnel: ["QnRtn=1" w319 "ExeRtn=1"] -> w315
        frame "返回请求应答", Default {
        }
        frame "上传数据" {
          n196 = global read "全局1.vi" "版本信息"() -> (w318:string)
          n197 = Concatenate Strings("Version=", w318) -> (w319:string)
        }
        frame "返回执行结果" {
        }
      }
    }
    frame "获取仪器软件版本号" {
      (unwired) ""
      n198 = global read "全局1.vi" "枚举"() -> (w323:enum16{"返回请求应答", "上传数据", "返回执行结果"})
      n199 = case shown="\"上传数据\"" w323 {
        tunnel: ["QnRtn=1" w329 "ExeRtn=1"] -> w322
        frame "返回请求应答", Default {
        }
        frame "上传数据" {
          n200 = global read "全局1.vi" "固件版本"() -> (w328:T7)
          n201 = global read "全局 小时数据发送次数.vi" "小时数据发送次数"() -> (w326:i32)
          n202 = Cluster To Array(cluster=w328) -> (array=w327:string[])
          n203 = Index Array(array=w327, index=w326) -> (element=w325:string)
          n204 = Concatenate Strings("FirmwareVersion=", w325) -> (w329:string)
        }
        frame "返回执行结果" {
        }
      }
    }
    frame "提取实时数据间隔" {
      (unwired) ""
      n205 = global read "全局1.vi" "枚举"() -> (w333:enum16{"返回请求应答", "上传数据", "返回执行结果"})
      n206 = case shown="\"上传数据\"" w333 {
        tunnel: ["QnRtn=1" w337 "ExeRtn=1"] -> w332
        frame "返回请求应答", Default {
        }
        frame "上传数据" {
          n207 = global read "实时数据发送间隔全局.vi" "实时数据发送间隔"() -> (w336:u32)
          n208 = Number To Decimal String(number=w336) -> (decimal integer string=w335:string)  [unwired: 1 in]
          n209 = Concatenate Strings("RtdInterval=", w335) -> (w337:string)
        }
        frame "返回执行结果" {
        }
      }
    }
    frame "实时数据" {
      # "包含质控数据主动上传"
      n210 = global read "全局 实时数据参数.vi" "实时数据参数"() -> (w342:string)
      n211 = case shown="\"集成干预测试\"" w342 {
        tunnel: [w346 w371 w396 w427 w451 w472] -> w343
        tunnel: w341 -> [w345 w370 w395 w425 w449 w470]
        tunnel: w340 -> [w344 w369 w394 w424 w448 w469]
        frame "水样测试", Default {
          n212 = global read "全局1.vi" "枚举"() -> (w347:enum16{"返回请求应答", "上传数据", "返回执行结果"})
          n213 = case shown="\"上传数据\"" w347 {
            tunnel: ["QnRtn=1" w365 "ExeRtn=1"] -> w346
            tunnel: w345 -> [_ w351 _]
            tunnel: w344 -> [_ w349 _]
            frame "返回请求应答", Default {
            }
            frame "上传数据" {
              n214 = call "数据发送组合-20200825 (子VI).vi"("枚举"=T4."实时数据", "插值后的数组元素"=w351) -> ("字符串"=w352:string)  [unwired: 9 in]
              n215 = global read "全局 小时数据发送次数.vi" "小时数据发送次数"() -> (w363:i32)
              n216 = Index Array(array=w349, index (row)=w363) -> (element=w362:string[])  [unwired: 1 in]
              n217 = Index Array(array=w362, index=0 ("索引")) -> (element=w360:string)
              n218 = call "规范时间戳.vi"("字符串"=w360) -> ("result string"=w358:string)  [unwired: 10 in]
              n219 = Empty String/Path?(string/path=w352) -> (empty?=w364:bool)
              n220 = Format Into String(format string="DataTime=%s;", w358) -> (resulting string=w357:string)  [unwired: 2 in, 1 out]
              n221 = Concatenate Strings(w357, w352) -> (w354:string)
              n222 = String Length(string=w354) -> (length=w356:i32)
              n223 = Decrement(x=w356) -> (x-1=w355:i32)
              n224 = String Subset(string=w354, length (rest)=w355) -> (substring=w353:string)  [unwired: 1 in]
              n225 = case shown="假" w364 {
                tunnel: [w366 ""] -> w365
                tunnel: w353 -> [w366 _]
                frame False {
                }
                frame True {
                }
              }
            }
            frame "返回执行结果" {
            }
          }
        }
        frame "平行样测试" {
          n226 = global read "全局1.vi" "枚举"() -> (w372:enum16{"返回请求应答", "上传数据", "返回执行结果"})
          n227 = case shown="\"上传数据\"" w372 {
            tunnel: ["QnRtn=1" w384 "ExeRtn=1"] -> w371
            tunnel: w369 -> [_ w378 _]
            tunnel: w370 -> [_ w375 _]
            frame "返回请求应答", Default {
            }
            frame "上传数据" {
              # "CODMn"
              n228 = call "数据发送组合-20200825 (子VI).vi"("枚举"=T4."平行样测试", "插值后的数组元素"=w375) -> ("字符串"=w374:string)  [unwired: 9 in]
              n229 = global read "全局 小时数据发送次数.vi" "小时数据发送次数"() -> (w377:i32)
              n230 = Index Array(array=w378, index (row)=w377) -> (element=w382:string[])  [unwired: 1 in]
              n231 = Index Array(array=w382, index=0 ("索引")) -> (element=w379:string)
              n232 = call "规范时间戳.vi"("字符串"=w379) -> ("result string"=w380:string)  [unwired: 10 in]
              n233 = Empty String/Path?(string/path=w379) -> (empty?=w383:bool)
              n234 = Format Into String(format string="DataTime=%s;%s" ("格式字符串"), w380, w374) -> (resulting string=w385:string)  [unwired: 2 in, 1 out]
              n235 = case shown="真" w383 {
                tunnel: [w389 ""] -> w384
                tunnel: w385 -> [w389 _]
                frame False {
                  n236 = global read "全局 小时数据发送次数.vi" "小时数据发送次数"() -> (w388:i32)
                  n237 = Increment(x=w388) -> (x+1=w387:i32)
                  n238 = global write "全局 小时数据发送次数.vi" "小时数据发送次数"(w387) -> ()
                }
                frame True {
                  n239 = global read "全局 小时数据发送次数.vi" "小时数据发送次数"() -> (w391:i32)
                  n240 = Increment(x=w391) -> (x+1=w390:i32)
                  n241 = global write "全局 小时数据发送次数.vi" "小时数据发送次数"(w390) -> ()
                }
              }
            }
            frame "返回执行结果" {
            }
          }
        }
        frame "集成干预测试" {
          n242 = global read "全局1.vi" "枚举"() -> (w397:enum16{"返回请求应答", "上传数据", "返回执行结果"})
          n243 = case shown="\"上传数据\"" w397 {
            tunnel: ["QnRtn=1" w410 "ExeRtn=1"] -> w396
            tunnel: w394 -> [_ w404 _]
            tunnel: w395 -> [_ w401 _]
            frame "返回请求应答", Default {
            }
            frame "上传数据" {
              # "CODMn"
              n244 = global read "全局 小时数据发送次数.vi" "小时数据发送次数"() -> (w403:i32)
              n245 = call "数据发送组合-20200825 (子VI).vi"("枚举"=T4."集成干预测试", "插值后的数组元素"=w401) -> ("字符串"=w400:string)  [unwired: 9 in]
              n246 = Index Array(array=w404, index (row)=w403) -> (element=w408:string[])  [unwired: 1 in]
              n247 = global read "断电保存全局.vi" "应用环境"() -> (w399:T8)
              n248 = Index Array(array=w408, index=0 ("索引")) -> (element=w405:string)
              n249 = case shown="\"GB212\", 默认" w399 {
                tunnel: [w414 w415] -> w406
                tunnel: w405 -> [w413 w416]
                frame "STD" {
                  n250 = call "规范时间戳.vi"("字符串"=w413) -> ("result string"=w414:string)  [unwired: 10 in]
                }
                frame "GB212", Default {
                  n251 = call "规范分钟数据时间戳.vi"("字符串"=w416) -> ("result string"=w415:string)  [unwired: 10 in]
                }
              }
              n252 = Empty String/Path?(string/path=w405) -> (empty?=w409:bool)
              n253 = Format Into String(format string="DataTime=%s;%s" ("格式字符串"), w406, w400) -> (resulting string=w411:string)  [unwired: 2 in, 1 out]
              n254 = case shown="假" w409 {
                tunnel: [w419 ""] -> w410
                tunnel: w411 -> [w419 _]
                frame False {
                  n255 = global read "全局 小时数据发送次数.vi" "小时数据发送次数"() -> (w418:i32)
                  n256 = Increment(x=w418) -> (x+1=w417:i32)
                  n257 = global write "全局 小时数据发送次数.vi" "小时数据发送次数"(w417) -> ()
                }
                frame True {
                  n258 = global read "全局 小时数据发送次数.vi" "小时数据发送次数"() -> (w421:i32)
                  n259 = Increment(x=w421) -> (x+1=w420:i32)
                  n260 = global write "全局 小时数据发送次数.vi" "小时数据发送次数"(w420) -> ()
                }
              }
            }
            frame "返回执行结果" {
            }
          }
        }
        frame "加标回收测试" {
          n261 = global read "全局1.vi" "枚举"() -> (w426:enum16{"返回请求应答", "上传数据", "返回执行结果"})
          n262 = case shown="\"上传数据\"" w426 {
            tunnel: ["QnRtn=1" w437 "ExeRtn=1"] -> w427
            tunnel: w424 -> [_ w432 _]
            tunnel: w425 -> [_ w434 _]
            frame "返回请求应答", Default {
            }
            frame "上传数据" {
              # "w01001-Check=63.0,w01001-WaterTime=20160801080000,w01001-Water=45.23,w01001-Chroma=1000,w01001-Volume=0.2,w01001-DVolume=200,w01003-Flag=N;"
              # "CODMn"
              n263 = global read "全局 小时数据发送次数.vi" "小时数据发送次数"() -> (w431:i32)
              n264 = call "加标回收数据组合 (子VI).vi"("小时数据发送次数"=w431, "数据"=w432, "污染物编码"="CODMn") -> ("datatime"=w430:string)  [unwired: 7 in, 1 out]
              n265 = call "规范时间戳.vi"("字符串"=w430) -> ("result string"=w439:string)  [unwired: 10 in]
              n266 = Empty String/Path?(string/path=w439) -> (empty?=w436:bool)
              n267 = call "数据发送组合-20200825 (子VI).vi"("枚举"=T4."加标回收测试", "插值后的数组元素"=w434) -> ("字符串"=w433:string)  [unwired: 9 in]
              n268 = Format Into String(format string="DataTime=%s;%s" ("格式字符串"), w439, w433) -> (resulting string=w438:string)  [unwired: 2 in, 1 out]
              n269 = case shown="真" w436 {
                tunnel: [w443 ""] -> w437
                tunnel: w438 -> [w443 _]
                frame False {
                  n270 = global read "全局 小时数据发送次数.vi" "小时数据发送次数"() -> (w442:i32)
                  n271 = Increment(x=w442) -> (x+1=w441:i32)
                  n272 = global write "全局 小时数据发送次数.vi" "小时数据发送次数"(w441) -> ()
                }
                frame True {
                  n273 = global read "全局 小时数据发送次数.vi" "小时数据发送次数"() -> (w445:i32)
                  n274 = Increment(x=w445) -> (x+1=w444:i32)
                  n275 = global write "全局 小时数据发送次数.vi" "小时数据发送次数"(w444) -> ()
                }
              }
            }
            frame "返回执行结果" {
            }
          }
        }
        frame "核查数据" {
          n276 = global read "全局1.vi" "枚举"() -> (w450:enum16{"返回请求应答", "上传数据", "返回执行结果"})
          n277 = case shown="\"上传数据\"" w450 {
            tunnel: ["QnRtn=1" w461 "ExeRtn=1"] -> w451
            tunnel: w449 -> [_ w454 _]
            tunnel: w448 -> [_ w453 _]
            frame "返回请求应答", Default {
            }
            frame "上传数据" {
              # "将非空数组的时间戳写入"
              n278 = global read "全局 小时数据发送次数.vi" "小时数据发送次数"() -> (w457:i32)
              n279 = Index Array(array=w453, index (row)=w457) -> (element=w460:string[])  [unwired: 1 in]
              n280 = call "数据发送组合-20200825 (子VI).vi"("枚举"=T4."核查数据", "插值后的数组元素"=w454) -> ("字符串"=w455:string)  [unwired: 9 in]
              n281 = Index Array(array=w460, index=0 ("索引")) -> (element=w459:string)
              n282 = call "规范分钟数据时间戳.vi"("字符串"=w459) -> ("result string"=w458:string)  [unwired: 10 in]
              n283 = Empty String/Path?(string/path=w458) -> (empty?=w463:bool)
              n284 = Format Into String(format string="DataTime=%s;%s" ("格式字符串"), w458, w455) -> (resulting string=w462:string)  [unwired: 2 in, 1 out]
              n285 = case shown="假" w463 {
                tunnel: [w466 ""] -> w461
                tunnel: w462 -> [w466 _]
                frame False {
                }
                frame True {
                }
              }
            }
            frame "返回执行结果" {
            }
          }
        }
        frame "空白测试", "跨度核查" {
          n286 = global read "全局1.vi" "枚举"() -> (w471:enum16{"返回请求应答", "上传数据", "返回执行结果"})
          n287 = case shown="\"上传数据\"" w471 {
            tunnel: ["QnRtn=1" w483 "ExeRtn=1"] -> w472
            tunnel: w470 -> [_ w479 _]
            tunnel: w469 -> [_ w477 _]
            frame "返回请求应答", Default {
            }
            frame "上传数据" {
              n288 = global read "全局 小时数据发送次数.vi" "小时数据发送次数"() -> (w481:i32)
              n289 = call "数据发送组合-20200825 (子VI).vi"("枚举"=T4."空白零点跨度数据", "插值后的数组元素"=w479) -> ("字符串"=w478:string)  [unwired: 9 in]
              n290 = Index Array(array=w477, index (row)=w481) -> (element=w487:string[])  [unwired: 1 in]
              n291 = Index Array(array=w487, index #1=0 ("索引"), index #2=3 ("索引"), index #3=5 ("索引")) -> (element #1=w475:string, element #3=w476:string)  [unwired: 1 out]
              n292 = case shown="\"pf\"" w476 {
                tunnel: [w490 w492] -> w474
                tunnel: w475 -> [w491 w493]
                frame "假", Default {
                  n293 = call "规范小时时间戳.vi"("字符串"=w491) -> ("result string"=w490:string)  [unwired: 10 in]
                }
                frame "pf" {
                  # "pf数据时间戳不变"
                  n294 = call "规范时间戳.vi"("字符串"=w493) -> ("result string"=w492:string)  [unwired: 10 in]
                }
              }
              n295 = Empty String/Path?(string/path=w474) -> (empty?=w484:bool)
              n296 = Format Into String(format string="DataTime=%s;%s" ("格式字符串"), w474, w478) -> (resulting string=w482:string)  [unwired: 2 in, 1 out]
              n297 = case shown="假" w484 {
                tunnel: [w494 ""] -> w483
                tunnel: w482 -> [w494 _]
                frame False {
                }
                frame True {
                }
              }
            }
            frame "返回执行结果" {
            }
          }
        }
      }
    }
    frame "小时数据" {
      # "发送小时数据"
      n298 = global read "全局1.vi" "枚举"() -> (w500:enum16{"返回请求应答", "上传数据", "返回执行结果"})
      n299 = case shown="\"上传数据\"" w500 {
        tunnel: ["QnRtn=1" w522 "ExeRtn=1"] -> w498
        tunnel: w499 -> [_ w510 _]
        tunnel: w497 -> [_ w507 _]
        frame "返回请求应答", Default {
          (unwired) 0 ("当前包数")
          n300 = global read "全局 数据数组大小.vi" "数据数组大小"() -> (w501:i32)
          n301 = global write "全局1.vi" "枚举"(enum16{"返回请求应答", "上传数据", "返回执行结果"}."上传数据" ("枚举")) -> ()
          n302 = Equal To 0?(x=w501) -> (x = 0?=w502:bool)
          n303 = case shown="真" w502 {
            frame False {
            }
            frame True {
              n304 = global read "全局 小时数据发送次数.vi" "小时数据发送次数"() -> (w506:i32)
              n305 = Increment(x=w506) -> (x+1=w505:i32)
              n306 = global write "全局 小时数据发送次数.vi" "小时数据发送次数"(w505) -> ()
            }
          }
        }
        frame "上传数据" {
          n307 = global read "全局 小时数据发送次数.vi" "小时数据发送次数"() -> (w521:i32)
          n308 = call "数据发送组合-20200825 (子VI).vi"("枚举"=enum16{"小时数据", "实时数据"}."小时数据", "插值后的数组元素"=w510) -> ("字符串"=w508:string)  [unwired: 9 in]
          n309 = Index Array(array=w507, index (row)=w521) -> (element=w520:string[])  [unwired: 1 in]
          n310 = Index Array(array=w520, index=0 ("索引")) -> (element=w518:string)
          n311 = call "规范小时时间戳.vi"("字符串"=w518) -> ("result string"=w515:string)  [unwired: 10 in]
          n312 = Empty String/Path?(string/path=w508) -> (empty?=w523:bool)
          n313 = Format Into String(format string="DataTime=%s;", w515) -> (resulting string=w517:string)  [unwired: 2 in, 1 out]
          n314 = Concatenate Strings(w517, w508) -> (w512:string)
          n315 = String Length(string=w512) -> (length=w514:i32)
          n316 = Decrement(x=w514) -> (x-1=w513:i32)
          n317 = String Subset(string=w512, length (rest)=w513) -> (substring=w511:string)  [unwired: 1 in]
          n318 = case shown="假" w523 {
            tunnel: [w524 ""] -> w522
            tunnel: w511 -> [w524 _]
            frame False {
            }
            frame True {
            }
          }
        }
        frame "返回执行结果" {
          (unwired) 0 ("当前包数")
          n319 = global write "全局1.vi" "枚举"(enum16{"返回请求应答", "上传数据", "返回执行结果"}."返回请求应答" ("枚举")) -> ()
        }
      }
    }
    frame "剖面数据" {
      # "{\"data\":[{\"time\":\"21-06-08 01:08:00\",\"w01010Value\":23,\"w01001Value\":7,\"w01009Value\":6,\"w01014Value\":22,\"w01003Value\":100,\"depth\":0.5,\"row\":3},{\"time\":\"21-06-08 01:08:00\",\"w01010Value\":22,\"w01001Value\":8,\"w01009Value\":7,\"w01014Value\":25,\"w01003Value\":96,\"depth\":0.8,\"row\":3},{\"time\":\"21-06-08 01:08:00\",\"w01010Value\":21,\"w01001Value\":7,\"w01009Value\":7,\"w01014Value\":24,\"w01003Value\":95,\"depth\":1,\"row\":3}]}"
      # "发送剖面数据"
      n320 = global read "全局1.vi" "枚举"() -> (w528:enum16{"返回请求应答", "上传数据", "返回执行结果"})
      n321 = case shown="\"上传数据\"" w528 {
        tunnel: ["QnRtn=1" w539 "ExeRtn=1"] -> w529
        frame "返回请求应答", Default {
          (unwired) 0 ("当前包数")
          n322 = global read "全局 数据数组大小.vi" "数据数组大小"() -> (w530:i32)
          n323 = global write "全局1.vi" "枚举"(enum16{"返回请求应答", "上传数据", "返回执行结果"}."上传数据" ("枚举")) -> ()
          n324 = Equal To 0?(x=w530) -> (x = 0?=w531:bool)
          n325 = case shown="真" w531 {
            frame False {
            }
            frame True {
              n326 = global read "全局 小时数据发送次数.vi" "小时数据发送次数"() -> (w535:i32)
              n327 = Increment(x=w535) -> (x+1=w534:i32)
              n328 = global write "全局 小时数据发送次数.vi" "小时数据发送次数"(w534) -> ()
            }
          }
        }
        frame "上传数据" {
          n329 = global read "断电保存全局.vi" "数据发送协议"() -> (w538:enum16{"2005-212协议", "2017-212协议"})
          n330 = case shown="\"2017-212协议\", 默认" w538 {
            tunnel: ["" ("编码输出") w560] -> w537
            tunnel: [_ w556] -> w536
            frame "2005-212协议" {
            }
            frame "2017-212协议", Default {
              w550 = 0 ("索引 (行)")
              (unwired) "w01010" ("污染物编码")
              (unwired) "w01016" ("污染物编码")
              (unwired) "w01003" ("污染物编码")
              (unwired) "w01014" ("污染物编码")
              # "时间,测量模式,数据类型,数据标识,层数,Temp,SpCond,Cond,Sal,TDS,pH,pHmV,ORP,ODO%,ODOmg/L,Turb,Chla,Depth,"
              n331 = global read "全局 小时数据发送次数.vi" "小时数据发送次数"() -> (w559:i32)
              n332 = global read "全局 所有参数.vi" "剖面多参数"() -> (w547:string[][])
              n333 = global read "全局 数据数组大小.vi" "分包标准"() -> (w558:i32)
              n334 = global read "全局 所有参数.vi" "columns"() -> (w557:string[])
              n335 = Array Subset(array=w547, index (row)=w559, length (row)=w558) -> (w556:string[][])  [unwired: 2 in]
              n336 = Array Subset(array=w547, index (row)=0 ("索引"), length (row)=1 ("长度")) -> (w545:string[][])  [unwired: 2 in]
              n337 = call "新剖面数据组合.vi"("columns"=w557, "剖面数据"=w556) -> ("结果字符串"=w554:string)  [unwired: 9 in]
              n338 = Index Array(array=w545, index (row) #1=w550, index (col) #1=0 ("索引 (行)"), index (row) #2=w550, index (col) #2=1 ("索引 (列)"), index (row) #3=w550, index (col) #3=2 ("索引 (列)")) -> (element #1=w543:string, element #2=w549:string, element #3=w548:string)
              n339 = call "规范小时时间戳.vi"("字符串"=w543) -> ("result string"=w542:string)  [unwired: 10 in]
              n340 = Empty String/Path?(string/path=w554) -> (empty?=w561:bool)
              n341 = Format Into String(format string="DataTime=%s;total=%s;waterdepth=%s;data=%s", w542, w549, w548, w554) -> (resulting string=w553:string)  [unwired: 2 in, 1 out]
              n342 = case shown="真" w561 {
                tunnel: [w563 ""] -> w560
                tunnel: w553 -> [w563 _]
                frame False {
                }
                frame True {
                }
              }
            }
          }
          n343 = Empty String/Path?(string/path=w537) -> (empty?=w540:bool)
          n344 = case shown="假" w540 {
            tunnel: [w570 ""] -> w539
            tunnel: w537 -> [w570 _]
            tunnel: w536 -> [w569 w571]
            frame False {
              n345 = Array Size(array=w569) -> (size(s)=w568:i32[])
              n346 = global read "全局 小时数据发送次数.vi" "小时数据发送次数"() -> (w566:i32)
              n347 = Index Array(array=w568) -> (element=w567:i32)  [unwired: 1 in]
              n348 = Add(x=w567, y=w566) -> (x+y=w565:i32)
              n349 = global write "全局 小时数据发送次数.vi" "小时数据发送次数"(w565) -> ()
            }
            frame True {
              n350 = Array Size(array=w571) -> (size(s)=w575:i32[])
              n351 = global read "全局 小时数据发送次数.vi" "小时数据发送次数"() -> (w573:i32)
              n352 = Index Array(array=w575) -> (element=w574:i32)  [unwired: 1 in]
              n353 = Add(x=w574, y=w573) -> (x+y=w572:i32)
              n354 = global write "全局 小时数据发送次数.vi" "小时数据发送次数"(w572) -> ()
            }
          }
        }
        frame "返回执行结果" {
          (unwired) 0 ("当前包数")
          n355 = global write "全局1.vi" "枚举"(enum16{"返回请求应答", "上传数据", "返回执行结果"}."返回请求应答" ("枚举")) -> ()
        }
      }
    }
    frame "剖面多参数H" {
      # "发送小时数据"
      n356 = global read "全局1.vi" "枚举"() -> (w579:enum16{"返回请求应答", "上传数据", "返回执行结果"})
      n357 = case shown="\"上传数据\"" w579 {
        tunnel: ["QnRtn=1" w589 "ExeRtn=1"] -> w580
        frame "返回请求应答", Default {
          (unwired) 0 ("当前包数")
          n358 = global read "全局 数据数组大小.vi" "数据数组大小"() -> (w581:i32)
          n359 = global write "全局1.vi" "枚举"(enum16{"返回请求应答", "上传数据", "返回执行结果"}."上传数据" ("枚举")) -> ()
          n360 = Equal To 0?(x=w581) -> (x = 0?=w582:bool)
          n361 = case shown="真" w582 {
            frame False {
            }
            frame True {
              n362 = global read "全局 小时数据发送次数.vi" "小时数据发送次数"() -> (w586:i32)
              n363 = Increment(x=w586) -> (x+1=w585:i32)
              n364 = global write "全局 小时数据发送次数.vi" "小时数据发送次数"(w585) -> ()
            }
          }
        }
        frame "上传数据" {
          n365 = global read "断电保存全局.vi" "数据发送协议"() -> (w588:enum16{"2005-212协议", "2017-212协议"})
          n366 = case shown="\"2017-212协议\", 默认" w588 {
            tunnel: ["" ("编码输出") w595] -> w587
            frame "2005-212协议" {
            }
            frame "2017-212协议", Default {
              (unwired) "w01010" ("污染物编码")
              (unwired) "w01016" ("污染物编码")
              (unwired) "w01003" ("污染物编码")
              (unwired) "w01009" ("污染物编码")
              (unwired) "w01001" ("污染物编码")
              (unwired) "w01014" ("污染物编码")
              (unwired) "w01100" ("污染物编码")
              # "时间,测量模式,数据类型,数据标识,层数,Temp,SpCond,Cond,Sal,TDS,pH,pHmV,ORP,ODO%,ODOmg/L,Turb,Chla,Depth,"
              n367 = global read "全局 小时数据发送次数.vi" "小时数据发送次数"() -> (w613:i32)
              n368 = global read "全局 所有参数.vi" "剖面多参数"() -> (w616:string[][])
              n369 = Index Array(array=w616, index (row)=w613) -> (element=w614:string[])  [unwired: 1 in]
              n370 = Index Array(array=w614, index #1=0 ("索引")) -> (element #1=w598:string, element #3=w612:string, element #4=w611:string, element #5=w610:string, element #6=w609:string, element #7=w608:string, element #11=w606:string, element #13=w605:string, element #15=w604:string, element #16=w603:string, element #17=w602:string, element #18=w592:string)  [unwired: 17 in, 6 out]
              n371 = call "规范小时时间戳.vi"("字符串"=w598) -> ("result string"=w599:string)  [unwired: 10 in]
              n372 = Build Array(w609, w608, w606, w605, w604, w603, w602, w592) -> (w607:string[])
              n373 = call "剖面多参数组合(子VI).vi"("数据类型实时小时"="-Avg=", "数据值"=w607, "层数"=w610, "数据标识"=w611, "数据类型"=w612) -> ("编码输出"=w594:string)  [unwired: 6 in]
              n374 = Format Into String(format string="DataTime=%s;", w599) -> (resulting string=w600:string)  [unwired: 2 in, 1 out]
              n375 = Empty String/Path?(string/path=w594) -> (empty?=w597:bool)
              n376 = Concatenate Strings(w600, w594) -> (w596:string)
              n377 = case shown="真" w597 {
                tunnel: [w617 ""] -> w595
                tunnel: w596 -> [w617 _]
                frame False {
                }
                frame True {
                }
              }
            }
          }
          n378 = Empty String/Path?(string/path=w587) -> (empty?=w590:bool)
          n379 = case shown="假" w590 {
            tunnel: [w621 ""] -> w589
            tunnel: w587 -> [w621 _]
            frame False {
              n380 = global read "全局 小时数据发送次数.vi" "小时数据发送次数"() -> (w620:i32)
              n381 = Increment(x=w620) -> (x+1=w619:i32)
              n382 = global write "全局 小时数据发送次数.vi" "小时数据发送次数"(w619) -> ()
            }
            frame True {
              n383 = global read "全局 小时数据发送次数.vi" "小时数据发送次数"() -> (w623:i32)
              n384 = Increment(x=w623) -> (x+1=w622:i32)
              n385 = global write "全局 小时数据发送次数.vi" "小时数据发送次数"(w622) -> ()
            }
          }
        }
        frame "返回执行结果" {
          (unwired) 0 ("当前包数")
          n386 = global write "全局1.vi" "枚举"(enum16{"返回请求应答", "上传数据", "返回执行结果"}."返回请求应答" ("枚举")) -> ()
        }
      }
    }
    frame "剖面多参数S" {
      # "发送实时数据"
      n387 = global read "全局1.vi" "枚举"() -> (w627:enum16{"返回请求应答", "上传数据", "返回执行结果"})
      n388 = case shown="\"上传数据\"" w627 {
        tunnel: ["QnRtn=1" w637 "ExeRtn=1"] -> w628
        frame "返回请求应答", Default {
          (unwired) 0 ("当前包数")
          n389 = global read "全局 数据数组大小.vi" "数据数组大小"() -> (w629:i32)
          n390 = global write "全局1.vi" "枚举"(enum16{"返回请求应答", "上传数据", "返回执行结果"}."上传数据" ("枚举")) -> ()
          n391 = Equal To 0?(x=w629) -> (x = 0?=w630:bool)
          n392 = case shown="真" w630 {
            frame False {
            }
            frame True {
              n393 = global read "全局 小时数据发送次数.vi" "小时数据发送次数"() -> (w634:i32)
              n394 = Increment(x=w634) -> (x+1=w633:i32)
              n395 = global write "全局 小时数据发送次数.vi" "小时数据发送次数"(w633) -> ()
            }
          }
        }
        frame "上传数据" {
          n396 = global read "断电保存全局.vi" "数据发送协议"() -> (w636:enum16{"2005-212协议", "2017-212协议"})
          n397 = case shown="\"2017-212协议\", 默认" w636 {
            tunnel: ["" ("编码输出") w645] -> w635
            frame "2005-212协议" {
            }
            frame "2017-212协议", Default {
              (unwired) "w01010" ("污染物编码")
              (unwired) "w01016" ("污染物编码")
              (unwired) "w01003" ("污染物编码")
              (unwired) "w01009" ("污染物编码")
              (unwired) "w01001" ("污染物编码")
              (unwired) "w01014" ("污染物编码")
              (unwired) "w01100" ("污染物编码")
              # "时间,测量模式,数据类型,数据标识,层数,Temp,SpCond,Cond,Sal,TDS,pH,pHmV,ORP,ODO%,ODOmg/L,Turb,Chla,Depth,"
              n398 = global read "全局 小时数据发送次数.vi" "小时数据发送次数"() -> (w661:i32)
              n399 = global read "全局 所有参数.vi" "剖面多参数"() -> (w664:string[][])
              n400 = Index Array(array=w664, index (row)=w661) -> (element=w662:string[])  [unwired: 1 in]
              n401 = Index Array(array=w662, index #1=0 ("索引")) -> (element #1=w642:string, element #3=w660:string, element #4=w659:string, element #5=w658:string, element #6=w657:string, element #7=w656:string, element #11=w654:string, element #13=w653:string, element #15=w652:string, element #16=w651:string, element #17=w650:string, element #18=w640:string)  [unwired: 17 in, 6 out]
              n402 = call "规范时间戳.vi"("字符串"=w642) -> ("result string"=w641:string)  [unwired: 10 in]
              n403 = Build Array(w657, w656, w654, w653, w652, w651, w650, w640) -> (w655:string[])
              n404 = call "剖面多参数组合(子VI).vi"("数据类型实时小时"="-Rtd=", "数据值"=w655, "层数"=w658, "数据标识"=w659, "数据类型"=w660) -> ("编码输出"=w644:string)  [unwired: 6 in]
              n405 = Format Into String(format string="DataTime=%s;", w641) -> (resulting string=w648:string)  [unwired: 2 in, 1 out]
              n406 = Empty String/Path?(string/path=w644) -> (empty?=w647:bool)
              n407 = Concatenate Strings(w648, w644) -> (w646:string)
              n408 = case shown="假" w647 {
                tunnel: [w665 ""] -> w645
                tunnel: w646 -> [w665 _]
                frame False {
                }
                frame True {
                }
              }
            }
          }
          n409 = Empty String/Path?(string/path=w635) -> (empty?=w638:bool)
          n410 = case shown="假" w638 {
            tunnel: [w669 ""] -> w637
            tunnel: w635 -> [w669 _]
            frame False {
              n411 = global read "全局 小时数据发送次数.vi" "小时数据发送次数"() -> (w668:i32)
              n412 = Increment(x=w668) -> (x+1=w667:i32)
              n413 = global write "全局 小时数据发送次数.vi" "小时数据发送次数"(w667) -> ()
            }
            frame True {
              n414 = global read "全局 小时数据发送次数.vi" "小时数据发送次数"() -> (w671:i32)
              n415 = Increment(x=w671) -> (x+1=w670:i32)
              n416 = global write "全局 小时数据发送次数.vi" "小时数据发送次数"(w670) -> ()
            }
          }
        }
        frame "返回执行结果" {
          (unwired) 0 ("当前包数")
          n417 = global write "全局1.vi" "枚举"(enum16{"返回请求应答", "上传数据", "返回执行结果"}."返回请求应答" ("枚举")) -> ()
        }
      }
    }
    frame "提取小时数据" {
      # "发送小时数据"
      n418 = global read "全局 小时数据发送次数.vi" "小时数据发送次数"() -> (w677:i32)
      n419 = Index Array(array=w679, index (row)=w677) -> (element=w676:string[])  [unwired: 1 in]
      n420 = global read "全局1.vi" "枚举"() -> (w678:enum16{"返回请求应答", "上传数据", "返回执行结果"})
      n421 = case shown="\"上传数据\"" w678 {
        tunnel: ["QnRtn=1" w694 "ExeRtn=1"] -> w680
        tunnel: w676 -> [_ w696 _]
        tunnel: w675 -> [_ w686 _]
        frame "返回请求应答", Default {
          n422 = global read "全局 数据数组大小.vi" "数据数组大小"() -> (w681:i32)
          n423 = Equal To 0?(x=w681) -> (x = 0?=w682:bool)
          n424 = case shown="真" w682 {
            frame False {
            }
            frame True {
              n425 = global read "全局 小时数据发送次数.vi" "小时数据发送次数"() -> (w685:i32)
              n426 = Increment(x=w685) -> (x+1=w684:i32)
              n427 = global write "全局 小时数据发送次数.vi" "小时数据发送次数"(w684) -> ()
            }
          }
        }
        frame "上传数据" {
          n428 = Index Array(array=w696, index #2=1 ("索引")) -> (element #1=w689:string)  [unwired: 1 in, 1 out]
          n429 = call "规范小时时间戳.vi"("字符串"=w689) -> ("result string"=w690:string)  [unwired: 10 in]
          n430 = call "数据发送组合-20200825 (子VI).vi"("枚举"=T4."提取小时数据", "插值后的数组元素"=w686) -> ("字符串"=w687:string)  [unwired: 9 in]
          n431 = Format Into String(format string="DataTime=%s;", w690) -> (resulting string=w693:string)  [unwired: 2 in, 1 out]
          n432 = Empty String/Path?(string/path=w687) -> (empty?=w695:bool)
          n433 = Concatenate Strings(w693, w687) -> (w691:string)
          n434 = case shown="假" w695 {
            tunnel: [w700 ""] -> w694
            tunnel: w691 -> [w700 _]
            frame False {
              n435 = global read "全局 小时数据发送次数.vi" "小时数据发送次数"() -> (w699:i32)
              n436 = Increment(x=w699) -> (x+1=w698:i32)
              n437 = global write "全局 小时数据发送次数.vi" "小时数据发送次数"(w698) -> ()
            }
            frame True {
              n438 = global read "全局 小时数据发送次数.vi" "小时数据发送次数"() -> (w702:i32)
              n439 = Increment(x=w702) -> (x+1=w701:i32)
              n440 = global write "全局 小时数据发送次数.vi" "小时数据发送次数"(w701) -> ()
            }
          }
        }
        frame "返回执行结果" {
        }
      }
    }
    frame "提取实时数据" {
      # "提取实时数据"
      n441 = global read "全局 小时数据发送次数.vi" "小时数据发送次数"() -> (w707:i32)
      n442 = Index Array(array=w710, index (row)=w707) -> (element=w706:string[])  [unwired: 1 in]
      n443 = global read "全局1.vi" "枚举"() -> (w708:enum16{"返回请求应答", "上传数据", "返回执行结果"})
      n444 = case shown="\"上传数据\"" w708 {
        tunnel: ["QnRtn=1" w719 "ExeRtn=1"] -> w709
        tunnel: w706 -> [_ w725 _]
        tunnel: w705 -> [_ w717 _]
        frame "返回请求应答", Default {
          n445 = global read "全局 数据数组大小.vi" "数据数组大小"() -> (w711:i32)
          n446 = Equal To 0?(x=w711) -> (x = 0?=w712:bool)
          n447 = case shown="真" w712 {
            frame False {
            }
            frame True {
              n448 = global read "全局 小时数据发送次数.vi" "小时数据发送次数"() -> (w715:i32)
              n449 = Increment(x=w715) -> (x+1=w714:i32)
              n450 = global write "全局 小时数据发送次数.vi" "小时数据发送次数"(w714) -> ()
            }
          }
        }
        frame "上传数据" {
          n451 = Index Array(array=w725, index #1=0 ("索引"), index #2=3 ("索引"), index #3=5 ("索引")) -> (element #1=w723:string)  [unwired: 2 out]
          n452 = call "规范时间戳.vi"("字符串"=w723) -> ("result string"=w722:string)  [unwired: 10 in]
          n453 = call "数据发送组合-20200825 (子VI).vi"("枚举"=T4."提取实时数据", "插值后的数组元素"=w717) -> ("字符串"=w716:string)  [unwired: 9 in]
          n454 = Empty String/Path?(string/path=w722) -> (empty?=w721:bool)
          n455 = Format Into String(format string="DataTime=%s;%s" ("格式字符串"), w722, w716) -> (resulting string=w720:string)  [unwired: 2 in, 1 out]
          n456 = case shown="真" w721 {
            tunnel: [w729 ""] -> w719
            tunnel: w720 -> [w729 _]
            frame False {
              n457 = global read "全局 小时数据发送次数.vi" "小时数据发送次数"() -> (w731:i32)
              n458 = Increment(x=w731) -> (x+1=w730:i32)
              n459 = global write "全局 小时数据发送次数.vi" "小时数据发送次数"(w730) -> ()
            }
            frame True {
              n460 = global read "全局 小时数据发送次数.vi" "小时数据发送次数"() -> (w733:i32)
              n461 = Increment(x=w733) -> (x+1=w732:i32)
              n462 = global write "全局 小时数据发送次数.vi" "小时数据发送次数"(w732) -> ()
            }
          }
        }
        frame "返回执行结果" {
        }
      }
    }
    frame "核查数据" {
      # "提取标样核查数据"
      n463 = global read "全局 小时数据发送次数.vi" "小时数据发送次数"() -> (w739:i32)
      n464 = Index Array(array=w736, index (row)=w739) -> (element=w738:string[])  [unwired: 1 in]
      n465 = global read "全局1.vi" "枚举"() -> (w740:enum16{"返回请求应答", "上传数据", "返回执行结果"})
      n466 = case shown="\"上传数据\"" w740 {
        tunnel: ["QnRtn=1" w752 "ExeRtn=1"] -> w741
        tunnel: w738 -> [_ w758 _]
        tunnel: w737 -> [_ w748 _]
        frame "返回请求应答", Default {
          n467 = global read "全局 数据数组大小.vi" "数据数组大小"() -> (w743:i32)
          n468 = Equal To 0?(x=w743) -> (x = 0?=w742:bool)
          n469 = case shown="真" w742 {
            frame False {
            }
            frame True {
              n470 = global read "全局 小时数据发送次数.vi" "小时数据发送次数"() -> (w746:i32)
              n471 = Increment(x=w746) -> (x+1=w745:i32)
              n472 = global write "全局 小时数据发送次数.vi" "小时数据发送次数"(w745) -> ()
            }
          }
        }
        frame "上传数据" {
          # "将非空数组的时间戳写入"
          n473 = Index Array(array=w758, index #1=0 ("索引"), index #2=3 ("索引"), index #3=6 ("索引")) -> (element #1=w751:string)  [unwired: 2 out]
          n474 = call "数据发送组合-20200825 (子VI).vi"("枚举"=T4."核查数据", "插值后的数组元素"=w748) -> ("字符串"=w747:string)  [unwired: 9 in]
          n475 = call "规范时间戳.vi"("字符串"=w751) -> ("result string"=w750:string)  [unwired: 10 in]
          n476 = Empty String/Path?(string/path=w750) -> (empty?=w754:bool)
          n477 = Format Into String(format string="DataTime=%s;%s" ("格式字符串"), w750, w747) -> (resulting string=w753:string)  [unwired: 2 in, 1 out]
          n478 = case shown="假" w754 {
            tunnel: [w762 ""] -> w752
            tunnel: w753 -> [w762 _]
            frame False {
              n479 = global read "全局 小时数据发送次数.vi" "小时数据发送次数"() -> (w761:i32)
              n480 = Increment(x=w761) -> (x+1=w760:i32)
              n481 = global write "全局 小时数据发送次数.vi" "小时数据发送次数"(w760) -> ()
            }
            frame True {
              n482 = global read "全局 小时数据发送次数.vi" "小时数据发送次数"() -> (w764:i32)
              n483 = Increment(x=w764) -> (x+1=w763:i32)
              n484 = global write "全局 小时数据发送次数.vi" "小时数据发送次数"(w763) -> ()
            }
          }
        }
        frame "返回执行结果" {
        }
      }
    }
    frame "空白测试", "跨度核查", "零点核查" {
      # "提取空白测试数据/零点核查数据/跨度核查数据"
      n485 = global read "全局 小时数据发送次数.vi" "小时数据发送次数"() -> (w770:i32)
      n486 = Index Array(array=w767, index (row)=w770) -> (element=w769:string[])  [unwired: 1 in]
      n487 = global read "全局1.vi" "枚举"() -> (w771:enum16{"返回请求应答", "上传数据", "返回执行结果"})
      n488 = case shown="\"上传数据\"" w771 {
        tunnel: ["QnRtn=1" w783 "ExeRtn=1"] -> w772
        tunnel: w769 -> [_ w788 _]
        tunnel: w768 -> [_ w779 _]
        frame "返回请求应答", Default {
          (unwired) 0 ("当前包数")
          n489 = global read "全局 数据数组大小.vi" "数据数组大小"() -> (w774:i32)
          n490 = Equal To 0?(x=w774) -> (x = 0?=w773:bool)
          n491 = case shown="真" w773 {
            frame False {
            }
            frame True {
              n492 = global read "全局 小时数据发送次数.vi" "小时数据发送次数"() -> (w777:i32)
              n493 = Increment(x=w777) -> (x+1=w776:i32)
              n494 = global write "全局 小时数据发送次数.vi" "小时数据发送次数"(w776) -> ()
            }
          }
        }
        frame "上传数据" {
          # "将非空数组的时间戳写入"
          n495 = Index Array(array=w788, index #1=0 ("索引"), index #2=3 ("索引")) -> (element #1=w782:string)  [unwired: 1 out]
          n496 = call "数据发送组合-20200825 (子VI).vi"("枚举"=T4."空白零点跨度数据", "插值后的数组元素"=w779) -> ("字符串"=w778:string)  [unwired: 9 in]
          n497 = call "规范时间戳.vi"("字符串"=w782) -> ("result string"=w781:string)  [unwired: 10 in]
          n498 = Empty String/Path?(string/path=w781) -> (empty?=w785:bool)
          n499 = Format Into String(format string="DataTime=%s;%s" ("格式字符串"), w781, w778) -> (resulting string=w784:string)  [unwired: 2 in, 1 out]
          n500 = case shown="假" w785 {
            tunnel: [w792 ""] -> w783
            tunnel: w784 -> [w792 _]
            frame False {
              n501 = global read "全局 小时数据发送次数.vi" "小时数据发送次数"() -> (w791:i32)
              n502 = Increment(x=w791) -> (x+1=w790:i32)
              n503 = global write "全局 小时数据发送次数.vi" "小时数据发送次数"(w790) -> ()
            }
            frame True {
              n504 = global read "全局 小时数据发送次数.vi" "小时数据发送次数"() -> (w794:i32)
              n505 = Increment(x=w794) -> (x+1=w793:i32)
              n506 = global write "全局 小时数据发送次数.vi" "小时数据发送次数"(w793) -> ()
            }
          }
        }
        frame "返回执行结果" {
        }
      }
    }
    frame "提取加标回收" {
      # "提取加标回收数据"
      n507 = global read "全局1.vi" "枚举"() -> (w800:enum16{"返回请求应答", "上传数据", "返回执行结果"})
      n508 = case shown="\"上传数据\"" w800 {
        tunnel: ["QnRtn=1" w812 "ExeRtn=1"] -> w798
        tunnel: w799 -> [_ w814 _]
        tunnel: w797 -> [_ w806 _]
        frame "返回请求应答", Default {
          n509 = global read "全局 数据数组大小.vi" "数据数组大小"() -> (w801:i32)
          n510 = Equal To 0?(x=w801) -> (x = 0?=w802:bool)
          n511 = case shown="真" w802 {
            frame False {
            }
            frame True {
              n512 = global read "全局 小时数据发送次数.vi" "小时数据发送次数"() -> (w805:i32)
              n513 = Increment(x=w805) -> (x+1=w804:i32)
              n514 = global write "全局 小时数据发送次数.vi" "小时数据发送次数"(w804) -> ()
            }
          }
        }
        frame "上传数据" {
          # "w01001-Check=63.0,w01001-WaterTime=20160801080000,w01001-Water=45.23,w01001-Chroma=1000,w01001-Volume=0.2,w01001-DVolume=200,w01003-Flag=N;"
          # "CODMn"
          n515 = global read "全局 小时数据发送次数.vi" "小时数据发送次数"() -> (w809:i32)
          n516 = call "数据发送组合-20200825 (子VI).vi"("枚举"=T4."加标回收测试", "插值后的数组元素"=w806) -> ("字符串"=w807:string)  [unwired: 9 in]
          n517 = call "加标回收数据组合 (子VI).vi"("小时数据发送次数"=w809, "数据"=w814, "污染物编码"="w01019") -> ("datatime"=w816:string)  [unwired: 7 in, 1 out]
          n518 = call "规范时间戳.vi"("字符串"=w816) -> ("result string"=w815:string)  [unwired: 10 in]
          n519 = Empty String/Path?(string/path=w815) -> (empty?=w811:bool)
          n520 = Format Into String(format string="DataTime=%s;%s" ("格式字符串"), w815, w807) -> (resulting string=w813:string)  [unwired: 2 in, 1 out]
          n521 = case shown="真" w811 {
            tunnel: [w820 ""] -> w812
            tunnel: w813 -> [w820 _]
            frame False {
              n522 = global read "全局 小时数据发送次数.vi" "小时数据发送次数"() -> (w819:i32)
              n523 = Increment(x=w819) -> (x+1=w818:i32)
              n524 = global write "全局 小时数据发送次数.vi" "小时数据发送次数"(w818) -> ()
            }
            frame True {
              n525 = global read "全局 小时数据发送次数.vi" "小时数据发送次数"() -> (w822:i32)
              n526 = Increment(x=w822) -> (x+1=w821:i32)
              n527 = global write "全局 小时数据发送次数.vi" "小时数据发送次数"(w821) -> ()
            }
          }
        }
        frame "返回执行结果" {
        }
      }
    }
    frame "提取平行样" {
      # "提取平行样数据"
      n528 = global read "全局1.vi" "枚举"() -> (w828:enum16{"返回请求应答", "上传数据", "返回执行结果"})
      n529 = case shown="\"上传数据\"" w828 {
        tunnel: ["QnRtn=1" w844 "ExeRtn=1"] -> w827
        tunnel: w826 -> [_ w838 _]
        tunnel: w825 -> [_ w834 _]
        frame "返回请求应答", Default {
          n530 = global read "全局 数据数组大小.vi" "数据数组大小"() -> (w829:i32)
          n531 = Equal To 0?(x=w829) -> (x = 0?=w830:bool)
          n532 = case shown="真" w830 {
            frame False {
            }
            frame True {
              n533 = global read "全局 小时数据发送次数.vi" "小时数据发送次数"() -> (w833:i32)
              n534 = Increment(x=w833) -> (x+1=w832:i32)
              n535 = global write "全局 小时数据发送次数.vi" "小时数据发送次数"(w832) -> ()
            }
          }
        }
        frame "上传数据" {
          # "CODMn"
          n536 = global read "全局 小时数据发送次数.vi" "小时数据发送次数"() -> (w837:i32)
          n537 = call "数据发送组合-20200825 (子VI).vi"("枚举"=T4."平行样测试", "插值后的数组元素"=w834) -> ("字符串"=w835:string)  [unwired: 9 in]
          n538 = Index Array(array=w838, index (row)=w837) -> (element=w842:string[])  [unwired: 1 in]
          n539 = Index Array(array=w842, index=0 ("索引")) -> (element=w839:string)
          n540 = call "规范时间戳.vi"("字符串"=w839) -> ("result string"=w840:string)  [unwired: 10 in]
          n541 = Empty String/Path?(string/path=w839) -> (empty?=w843:bool)
          n542 = Format Into String(format string="DataTime=%s;%s" ("格式字符串"), w840, w835) -> (resulting string=w845:string)  [unwired: 2 in, 1 out]
          n543 = case shown="真" w843 {
            tunnel: [w849 ""] -> w844
            tunnel: w845 -> [w849 _]
            frame False {
              n544 = global read "全局 小时数据发送次数.vi" "小时数据发送次数"() -> (w848:i32)
              n545 = Increment(x=w848) -> (x+1=w847:i32)
              n546 = global write "全局 小时数据发送次数.vi" "小时数据发送次数"(w847) -> ()
            }
            frame True {
              n547 = global read "全局 小时数据发送次数.vi" "小时数据发送次数"() -> (w851:i32)
              n548 = Increment(x=w851) -> (x+1=w850:i32)
              n549 = global write "全局 小时数据发送次数.vi" "小时数据发送次数"(w850) -> ()
            }
          }
        }
        frame "返回执行结果" {
        }
      }
    }
    frame "提取集成干预" {
      # "提取平行样数据"
      n550 = global read "全局1.vi" "枚举"() -> (w857:enum16{"返回请求应答", "上传数据", "返回执行结果"})
      n551 = case shown="\"上传数据\"" w857 {
        tunnel: ["QnRtn=1" w874 "ExeRtn=1"] -> w856
        tunnel: w855 -> [_ w869 _]
        tunnel: w854 -> [_ w866 _]
        frame "返回请求应答", Default {
          n552 = global read "全局 数据数组大小.vi" "数据数组大小"() -> (w858:i32)
          n553 = Equal To 0?(x=w858) -> (x = 0?=w859:bool)
          n554 = case shown="真" w859 {
            frame False {
            }
            frame True {
              n555 = global read "全局 小时数据发送次数.vi" "小时数据发送次数"() -> (w862:i32)
              n556 = Increment(x=w862) -> (x+1=w861:i32)
              n557 = global write "全局 小时数据发送次数.vi" "小时数据发送次数"(w861) -> ()
            }
          }
        }
        frame "上传数据" {
          # "CODMn"
          n558 = global read "全局 小时数据发送次数.vi" "小时数据发送次数"() -> (w870:i32)
          n559 = call "数据发送组合-20200825 (子VI).vi"("枚举"=T4."集成干预测试", "插值后的数组元素"=w866) -> ("字符串"=w867:string)  [unwired: 9 in]
          n560 = Index Array(array=w869, index (row)=w870) -> (element=w872:string[])  [unwired: 1 in]
          n561 = global read "断电保存全局.vi" "应用环境"() -> (w865:T8)
          n562 = Index Array(array=w872, index=0 ("索引")) -> (element=w864:string)
          n563 = case shown="\"GB212\", 默认" w865 {
            tunnel: [w878 w879] -> w863
            tunnel: w864 -> [w877 w880]
            frame "STD" {
              n564 = call "规范时间戳.vi"("字符串"=w877) -> ("result string"=w878:string)  [unwired: 10 in]
            }
            frame "GB212", Default {
              n565 = call "规范分钟数据时间戳.vi"("字符串"=w880) -> ("result string"=w879:string)  [unwired: 10 in]
            }
          }
          n566 = Empty String/Path?(string/path=w864) -> (empty?=w873:bool)
          n567 = Format Into String(format string="DataTime=%s;%s" ("格式字符串"), w863, w867) -> (resulting string=w875:string)  [unwired: 2 in, 1 out]
          n568 = case shown="真" w873 {
            tunnel: [w883 ""] -> w874
            tunnel: w875 -> [w883 _]
            frame False {
              n569 = global read "全局 小时数据发送次数.vi" "小时数据发送次数"() -> (w882:i32)
              n570 = Increment(x=w882) -> (x+1=w881:i32)
              n571 = global write "全局 小时数据发送次数.vi" "小时数据发送次数"(w881) -> ()
            }
            frame True {
              n572 = global read "全局 小时数据发送次数.vi" "小时数据发送次数"() -> (w885:i32)
              n573 = Increment(x=w885) -> (x+1=w884:i32)
              n574 = global write "全局 小时数据发送次数.vi" "小时数据发送次数"(w884) -> ()
            }
          }
        }
        frame "返回执行结果" {
        }
      }
    }
    frame "操作日志" {
      n575 = global read "全局 小时数据发送次数.vi" "小时数据发送次数"() -> (w890:i32)
      n576 = Index Array(array=w892, index (row)=w890) -> (element=w889:string[])  [unwired: 1 in]
      n577 = global read "全局1.vi" "枚举"() -> (w891:enum16{"返回请求应答", "上传数据", "返回执行结果"})
      n578 = case shown="\"上传数据\"" w891 {
        tunnel: ["QnRtn=1" w910 "ExeRtn=1"] -> w893
        tunnel: w889 -> [_ w912 _]
        tunnel: w888 -> [_ w900 _]
        frame "返回请求应答", Default {
          n579 = global read "全局 数据数组大小.vi" "数据数组大小"() -> (w896:i32)
          n580 = Equal To 0?(x=w896) -> (x = 0?=w895:bool)
          n581 = case shown="真" w895 {
            frame False {
            }
            frame True {
              n582 = global read "全局 小时数据发送次数.vi" "小时数据发送次数"() -> (w898:i32)
              n583 = Increment(x=w898) -> (x+1=w897:i32)
              n584 = global write "全局 小时数据发送次数.vi" "小时数据发送次数"(w897) -> ()
            }
          }
        }
        frame "上传数据" {
          n585 = Index Array(array=w912, index #1=0 ("索引"), index #2=2 ("索引")) -> (element #1=w905:string)  [unwired: 1 out]
          n586 = call "规范时间戳.vi"("字符串"=w905) -> ("result string"=w903:string)  [unwired: 10 in]
          n587 = call "数据发送组合-20200825 (子VI).vi"("枚举"=T5."操作日志", "插值后的数组元素"=w900) -> ("字符串"=w899:string)  [unwired: 9 in]
          n588 = Format Into String(format string="DataTime=%s;", w903) -> (resulting string=w902:string)  [unwired: 2 in, 1 out]
          n589 = Concatenate Strings(w902, w899) -> (w907:string)
          n590 = Empty String/Path?(string/path=w907) -> (empty?=w911:bool)
          n591 = String Length(string=w907) -> (length=w909:i32)
          n592 = Decrement(x=w909) -> (x-1=w908:i32)
          n593 = String Subset(string=w907, length (rest)=w908) -> (substring=w906:string)  [unwired: 1 in]
          n594 = case shown="假" w911 {
            tunnel: [w917 ""] -> w910
            tunnel: w906 -> [w917 _]
            frame False {
              n595 = global read "全局 小时数据发送次数.vi" "小时数据发送次数"() -> (w916:i32)
              n596 = Increment(x=w916) -> (x+1=w915:i32)
              n597 = global write "全局 小时数据发送次数.vi" "小时数据发送次数"(w915) -> ()
            }
            frame True {
              n598 = global read "全局 小时数据发送次数.vi" "小时数据发送次数"() -> (w919:i32)
              n599 = Increment(x=w919) -> (x+1=w918:i32)
              n600 = global write "全局 小时数据发送次数.vi" "小时数据发送次数"(w918) -> ()
            }
          }
        }
        frame "返回执行结果" {
        }
      }
    }
    frame "3092日志信息" {
      n601 = global read "全局 小时数据发送次数.vi" "小时数据发送次数"() -> (w924:i32)
      n602 = global read "全局 所有参数.vi" "CODMn"() -> (w922:string[][])
      n603 = Index Array(array=w922, index (row)=w924) -> (element=w923:string[])  [unwired: 1 in]
      n604 = global read "全局1.vi" "枚举"() -> (w925:enum16{"返回请求应答", "上传数据", "返回执行结果"})
      n605 = case shown="\"上传数据\"" w925 {
        tunnel: ["QnRtn=1" w944 "ExeRtn=1"] -> w926
        tunnel: w923 -> [_ w946 _]
        frame "返回请求应答", Default {
          n606 = global read "全局 数据数组大小.vi" "数据数组大小"() -> (w929:i32)
          n607 = Equal To 0?(x=w929) -> (x = 0?=w928:bool)
          n608 = case shown="真" w928 {
            frame False {
            }
            frame True {
              n609 = global read "全局 小时数据发送次数.vi" "小时数据发送次数"() -> (w931:i32)
              n610 = Increment(x=w931) -> (x+1=w930:i32)
              n611 = global write "全局 小时数据发送次数.vi" "小时数据发送次数"(w930) -> ()
            }
          }
        }
        frame "上传数据" {
          n612 = Index Array(array=w946, index #1=0 ("索引")) -> (element #1=w939:string, element #2=w932:string, element #3=w934:string)  [unwired: 2 in]
          n613 = Empty String/Path?(string/path=w932) -> (empty?=w945:bool)
          n614 = call "规范时间戳.vi"("字符串"=w939) -> ("result string"=w936:string)  [unwired: 10 in]
          n615 = Format Into String(format string="DataTime=%s;", w936) -> (resulting string=w937:string)  [unwired: 2 in, 1 out]
          n616 = Format Into String(format string="parameter=//%s//,content==//%s//;" ("格式字符串"), w932, w934) -> (resulting string=w933:string)  [unwired: 2 in, 1 out]
          n617 = Concatenate Strings(w937, w933) -> (w941:string)
          n618 = String Length(string=w941) -> (length=w943:i32)
          n619 = Decrement(x=w943) -> (x-1=w942:i32)
          n620 = String Subset(string=w941, length (rest)=w942) -> (substring=w940:string)  [unwired: 1 in]
          n621 = case shown="假" w945 {
            tunnel: [w950 ""] -> w944
            tunnel: w940 -> [w950 _]
            frame False {
              n622 = global read "全局 小时数据发送次数.vi" "小时数据发送次数"() -> (w949:i32)
              n623 = Increment(x=w949) -> (x+1=w948:i32)
              n624 = global write "全局 小时数据发送次数.vi" "小时数据发送次数"(w948) -> ()
            }
            frame True {
              n625 = global read "全局 小时数据发送次数.vi" "小时数据发送次数"() -> (w952:i32)
              n626 = Increment(x=w952) -> (x+1=w951:i32)
              n627 = global write "全局 小时数据发送次数.vi" "小时数据发送次数"(w951) -> ()
            }
          }
        }
        frame "返回执行结果" {
        }
      }
    }
    frame "3093报警信息" {
      n628 = global read "全局 小时数据发送次数.vi" "小时数据发送次数"() -> (w957:i32)
      n629 = global read "全局 所有参数.vi" "CODMn"() -> (w955:string[][])
      n630 = Index Array(array=w955, index (row)=w957) -> (element=w956:string[])  [unwired: 1 in]
      n631 = global read "全局1.vi" "枚举"() -> (w958:enum16{"返回请求应答", "上传数据", "返回执行结果"})
      n632 = case shown="\"上传数据\"" w958 {
        tunnel: ["QnRtn=1" w980 "ExeRtn=1"] -> w959
        tunnel: w956 -> [_ w982 _]
        frame "返回请求应答", Default {
          n633 = global read "全局 数据数组大小.vi" "数据数组大小"() -> (w962:i32)
          n634 = Equal To 0?(x=w962) -> (x = 0?=w961:bool)
          n635 = case shown="真" w961 {
            frame False {
            }
            frame True {
              n636 = global read "全局 小时数据发送次数.vi" "小时数据发送次数"() -> (w964:i32)
              n637 = Increment(x=w964) -> (x+1=w963:i32)
              n638 = global write "全局 小时数据发送次数.vi" "小时数据发送次数"(w963) -> ()
            }
          }
        }
        frame "上传数据" {
          n639 = Index Array(array=w982, index #1=0 ("索引")) -> (element #1=w975:string, element #2=w969:string, element #3=w968:string, element #5=w967:string, element #6=w966:string)  [unwired: 5 in, 1 out]
          n640 = case shown="\"产生\"" w966 {
            tunnel: ["0" "1"] -> w965
            frame "消除", Default {
            }
            frame "产生" {
            }
          }
          n641 = Empty String/Path?(string/path=w969) -> (empty?=w981:bool)
          n642 = call "规范时间戳.vi"("字符串"=w975) -> ("result string"=w972:string)  [unwired: 10 in]
          n643 = Format Into String(format string="DataTime=%s;", w972) -> (resulting string=w973:string)  [unwired: 2 in, 1 out]
          n644 = Format Into String(format string="parameter=//%s//,code=//%s//,content=//%s//,state=%s;" ("格式字符串"), w969, w967, w968, w965) -> (resulting string=w970:string)  [unwired: 2 in, 1 out]
          n645 = Concatenate Strings(w973, w970) -> (w977:string)
          n646 = String Length(string=w977) -> (length=w979:i32)
          n647 = Decrement(x=w979) -> (x-1=w978:i32)
          n648 = String Subset(string=w977, length (rest)=w978) -> (substring=w976:string)  [unwired: 1 in]
          n649 = case shown="假" w981 {
            tunnel: [w988 ""] -> w980
            tunnel: w976 -> [w988 _]
            frame False {
              n650 = global read "全局 小时数据发送次数.vi" "小时数据发送次数"() -> (w987:i32)
              n651 = Increment(x=w987) -> (x+1=w986:i32)
              n652 = global write "全局 小时数据发送次数.vi" "小时数据发送次数"(w986) -> ()
            }
            frame True {
              n653 = global read "全局 小时数据发送次数.vi" "小时数据发送次数"() -> (w990:i32)
              n654 = Increment(x=w990) -> (x+1=w989:i32)
              n655 = global write "全局 小时数据发送次数.vi" "小时数据发送次数"(w989) -> ()
            }
          }
        }
        frame "返回执行结果" {
        }
      }
    }
    frame "仪器参数" {
      n656 = case shown="\"氨氮\"" w996 {
        selector: w996 -> [w1000 _ _ _ _ _ _ _ _ _ _ _ _ _ _ _ _ _ _ _ _ _ _ _ _ _ _ _ _ _ _ _]
        tunnel: [w1000 w1003 w1007 w1011 w1015 w1019 w1023 w1027 w1031 w1035 w1039 w1043 w1047 w1051 w1055 w1059 w1063 w1067 w1071 w1075 w1079 w1083 w1087 w1091 w1095 w1099 w1103 w1107 w1111 w1115 w1119 w1123] -> w995
        tunnel: [1.0 ("风向") w1001 w1005 w1009 w1013 w1017 w1021 w1025 w1029 w1033 w1037 w1041 w1045 w1049 w1053 w1057 w1061 w1065 w1069 w1073 w1077 w1081 w1085 w1089 w1093 w1097 w1101 w1105 w1109 w1113 w1117 w1121] -> _
        frame "假", Default {
        }
        frame "CODMn" {
          n657 = global read "断电保存全局.vi" "参数系数簇"() -> (w1002:T9)
          n658 = global read "断电保存全局.vi" "因子编码簇"() -> (w1004:T10)
          n659 = Unbundle By Name(w1002) -> ("CODMn"=w1001:dbl)
          n660 = Unbundle By Name(w1004) -> ("CODMn"=w1003:string)
        }
        frame "CODCr" {
          n661 = global read "断电保存全局.vi" "参数系数簇"() -> (w1006:T9)
          n662 = global read "断电保存全局.vi" "因子编码簇"() -> (w1008:T10)
          n663 = Unbundle By Name(w1006) -> ("CODCr"=w1005:dbl)
          n664 = Unbundle By Name(w1008) -> ("CODCr"=w1007:string)
        }
        frame "DO" {
          n665 = global read "断电保存全局.vi" "参数系数簇"() -> (w1010:T9)
          n666 = global read "断电保存全局.vi" "因子编码簇"() -> (w1012:T10)
          n667 = Unbundle By Name(w1010) -> ("DO"=w1009:dbl)
          n668 = Unbundle By Name(w1012) -> ("DO"=w1011:string)
        }
        frame "铜" {
          n669 = global read "断电保存全局.vi" "参数系数簇"() -> (w1014:T9)
          n670 = global read "断电保存全局.vi" "因子编码簇"() -> (w1016:T10)
          n671 = Unbundle By Name(w1014) -> ("铜"=w1013:dbl)
          n672 = Unbundle By Name(w1016) -> ("铜"=w1015:string)
        }
        frame "PH" {
          n673 = global read "断电保存全局.vi" "参数系数簇"() -> (w1018:T9)
          n674 = global read "断电保存全局.vi" "因子编码簇"() -> (w1020:T10)
          n675 = Unbundle By Name(w1018) -> ("PH"=w1017:dbl)
          n676 = Unbundle By Name(w1020) -> ("PH"=w1019:string)
        }
        frame "氨氮" {
          n677 = global read "断电保存全局.vi" "参数系数簇"() -> (w1022:T9)
          n678 = global read "断电保存全局.vi" "因子编码簇"() -> (w1024:T10)
          n679 = Unbundle By Name(w1022) -> ("氨氮"=w1021:dbl)
          n680 = Unbundle By Name(w1024) -> ("氨氮"=w1023:string)
        }
        frame "比电导率" {
          n681 = global read "断电保存全局.vi" "参数系数簇"() -> (w1026:T9)
          n682 = global read "断电保存全局.vi" "因子编码簇"() -> (w1028:T10)
          n683 = Unbundle By Name(w1026) -> ("比电导率"=w1025:dbl)
          n684 = Unbundle By Name(w1028) -> ("比电导率"=w1027:string)
        }
        frame "水温" {
          n685 = global read "断电保存全局.vi" "参数系数簇"() -> (w1030:T9)
          n686 = global read "断电保存全局.vi" "因子编码簇"() -> (w1032:T10)
          n687 = Unbundle By Name(w1030) -> ("水温"=w1029:dbl)
          n688 = Unbundle By Name(w1032) -> ("水温"=w1031:string)
        }
        frame "COD" {
          n689 = global read "断电保存全局.vi" "参数系数簇"() -> (w1034:T9)
          n690 = global read "断电保存全局.vi" "因子编码簇"() -> (w1036:T10)
          n691 = Unbundle By Name(w1034) -> ("COD"=w1033:dbl)
          n692 = Unbundle By Name(w1036) -> ("COD"=w1035:string)
        }
        frame "浊度" {
          n693 = global read "断电保存全局.vi" "参数系数簇"() -> (w1038:T9)
          n694 = global read "断电保存全局.vi" "因子编码簇"() -> (w1040:T10)
          n695 = Unbundle By Name(w1038) -> ("浊度"=w1037:dbl)
          n696 = Unbundle By Name(w1040) -> ("浊度"=w1039:string)
        }
        frame "总氮" {
          n697 = global read "断电保存全局.vi" "参数系数簇"() -> (w1042:T9)
          n698 = global read "断电保存全局.vi" "因子编码簇"() -> (w1044:T10)
          n699 = Unbundle By Name(w1042) -> ("总氮"=w1041:dbl)
          n700 = Unbundle By Name(w1044) -> ("总氮"=w1043:string)
        }
        frame "总磷" {
          n701 = global read "断电保存全局.vi" "参数系数簇"() -> (w1046:T9)
          n702 = global read "断电保存全局.vi" "因子编码簇"() -> (w1048:T10)
          n703 = Unbundle By Name(w1046) -> ("总磷"=w1045:dbl)
          n704 = Unbundle By Name(w1048) -> ("总磷"=w1047:string)
        }
        frame "叶绿素a" {
          n705 = global read "断电保存全局.vi" "参数系数簇"() -> (w1050:T9)
          n706 = global read "断电保存全局.vi" "因子编码簇"() -> (w1052:T10)
          n707 = Unbundle By Name(w1050) -> ("叶绿素a"=w1049:dbl)
          n708 = Unbundle By Name(w1052) -> ("叶绿素a"=w1051:string)
        }
        frame "藻密度" {
          n709 = global read "断电保存全局.vi" "参数系数簇"() -> (w1054:T9)
          n710 = global read "断电保存全局.vi" "因子编码簇"() -> (w1056:T10)
          n711 = Unbundle By Name(w1054) -> ("藻密度"=w1053:dbl)
          n712 = Unbundle By Name(w1056) -> ("藻密度"=w1055:string)
        }
        frame "水位" {
          n713 = global read "断电保存全局.vi" "参数系数簇"() -> (w1058:T9)
          n714 = global read "断电保存全局.vi" "因子编码簇"() -> (w1060:T10)
          n715 = Unbundle By Name(w1058) -> ("水位"=w1057:dbl)
          n716 = Unbundle By Name(w1060) -> ("水位"=w1059:string)
        }
        frame "流速" {
          n717 = global read "断电保存全局.vi" "参数系数簇"() -> (w1062:T9)
          n718 = global read "断电保存全局.vi" "因子编码簇"() -> (w1064:T10)
          n719 = Unbundle By Name(w1062) -> ("流速"=w1061:dbl)
          n720 = Unbundle By Name(w1064) -> ("流速"=w1063:string)
        }
        frame "瞬时流量" {
          n721 = global read "断电保存全局.vi" "参数系数簇"() -> (w1066:T9)
          n722 = global read "断电保存全局.vi" "因子编码簇"() -> (w1068:T10)
          n723 = Unbundle By Name(w1066) -> ("瞬时流量"=w1065:dbl)
          n724 = Unbundle By Name(w1068) -> ("瞬时流量"=w1067:string)
        }
        frame "累积流量" {
          n725 = global read "断电保存全局.vi" "参数系数簇"() -> (w1070:T9)
          n726 = global read "断电保存全局.vi" "因子编码簇"() -> (w1072:T10)
          n727 = Unbundle By Name(w1070) -> ("累积流量"=w1069:dbl)
          n728 = Unbundle By Name(w1072) -> ("累积流量"=w1071:string)
        }
        frame "亚硝酸盐" {
          n729 = global read "断电保存全局.vi" "参数系数簇"() -> (w1074:T9)
          n730 = global read "断电保存全局.vi" "因子编码簇"() -> (w1076:T10)
          n731 = Unbundle By Name(w1074) -> ("亚硝酸盐"=w1073:dbl)
          n732 = Unbundle By Name(w1076) -> ("亚硝酸盐"=w1075:string)
        }
        frame "硫化物" {
          n733 = global read "断电保存全局.vi" "参数系数簇"() -> (w1078:T9)
          n734 = global read "断电保存全局.vi" "因子编码簇"() -> (w1080:T10)
          n735 = Unbundle By Name(w1078) -> ("硫化物"=w1077:dbl)
          n736 = Unbundle By Name(w1080) -> ("硫化物"=w1079:string)
        }
        frame "ORP" {
          n737 = global read "断电保存全局.vi" "参数系数簇"() -> (w1082:T9)
          n738 = global read "断电保存全局.vi" "因子编码簇"() -> (w1084:T10)
          n739 = Unbundle By Name(w1082) -> ("ORP"=w1081:dbl)
          n740 = Unbundle By Name(w1084) -> ("ORP"=w1083:string)
        }
        frame "铅" {
          n741 = global read "断电保存全局.vi" "参数系数簇"() -> (w1086:T9)
          n742 = global read "断电保存全局.vi" "因子编码簇"() -> (w1088:T10)
          n743 = Unbundle By Name(w1086) -> ("铅"=w1085:dbl)
          n744 = Unbundle By Name(w1088) -> ("铅"=w1087:string)
        }
        frame "镉" {
          n745 = global read "断电保存全局.vi" "参数系数簇"() -> (w1090:T9)
          n746 = global read "断电保存全局.vi" "因子编码簇"() -> (w1092:T10)
          n747 = Unbundle By Name(w1090) -> ("镉"=w1089:dbl)
          n748 = Unbundle By Name(w1092) -> ("镉"=w1091:string)
        }
        frame "锌" {
          n749 = global read "断电保存全局.vi" "参数系数簇"() -> (w1094:T9)
          n750 = global read "断电保存全局.vi" "因子编码簇"() -> (w1096:T10)
          n751 = Unbundle By Name(w1094) -> ("锌"=w1093:dbl)
          n752 = Unbundle By Name(w1096) -> ("锌"=w1095:string)
        }
        frame "镍" {
          n753 = global read "断电保存全局.vi" "参数系数簇"() -> (w1098:T9)
          n754 = global read "断电保存全局.vi" "因子编码簇"() -> (w1100:T10)
          n755 = Unbundle By Name(w1098) -> ("镍"=w1097:dbl)
          n756 = Unbundle By Name(w1100) -> ("镍"=w1099:string)
        }
        frame "锰" {
          n757 = global read "断电保存全局.vi" "参数系数簇"() -> (w1102:T9)
          n758 = global read "断电保存全局.vi" "因子编码簇"() -> (w1104:T10)
          n759 = Unbundle By Name(w1102) -> ("锰"=w1101:dbl)
          n760 = Unbundle By Name(w1104) -> ("锰"=w1103:string)
        }
        frame "汞" {
          n761 = global read "断电保存全局.vi" "参数系数簇"() -> (w1106:T9)
          n762 = global read "断电保存全局.vi" "因子编码簇"() -> (w1108:T10)
          n763 = Unbundle By Name(w1106) -> ("汞"=w1105:dbl)
          n764 = Unbundle By Name(w1108) -> ("汞"=w1107:string)
        }
        frame "气温" {
          n765 = global read "断电保存全局.vi" "参数系数簇"() -> (w1110:T9)
          n766 = global read "断电保存全局.vi" "因子编码簇"() -> (w1112:T10)
          n767 = Unbundle By Name(w1110) -> ("气温"=w1109:dbl)
          n768 = Unbundle By Name(w1112) -> ("气温"=w1111:string)
        }
        frame "气压" {
          n769 = global read "断电保存全局.vi" "参数系数簇"() -> (w1114:T9)
          n770 = global read "断电保存全局.vi" "因子编码簇"() -> (w1116:T10)
          n771 = Unbundle By Name(w1114) -> ("气压"=w1113:dbl)
          n772 = Unbundle By Name(w1116) -> ("气压"=w1115:string)
        }
        frame "风速" {
          n773 = global read "断电保存全局.vi" "参数系数簇"() -> (w1118:T9)
          n774 = global read "断电保存全局.vi" "因子编码簇"() -> (w1120:T10)
          n775 = Unbundle By Name(w1118) -> ("风速"=w1117:dbl)
          n776 = Unbundle By Name(w1120) -> ("风速"=w1119:string)
        }
        frame "风向" {
          n777 = global read "断电保存全局.vi" "参数系数簇"() -> (w1122:T9)
          n778 = global read "断电保存全局.vi" "因子编码簇"() -> (w1124:T10)
          n779 = Unbundle By Name(w1122) -> ("风向"=w1121:dbl)
          n780 = Unbundle By Name(w1124) -> ("风向"=w1123:string)
        }
      }
      n781 = global read "全局1.vi" "枚举"() -> (w997:enum16{"返回请求应答", "上传数据", "返回执行结果"})
      n782 = case shown="\"上传数据\"" w997 {
        tunnel: ["QnRtn=1" w1142 "ExeRtn=1"] -> w998
        tunnel: w994 -> [_ w1134 _]
        tunnel: w995 -> [_ w1133 _]
        tunnel: w993 -> [_ w1131 _]
        frame "返回请求应答", Default {
          n783 = global read "全局 数据数组大小.vi" "数据数组大小"() -> (w1127:i32)
          n784 = Equal To 0?(x=w1127) -> (x = 0?=w1126:bool)
          n785 = case shown="真" w1126 {
            frame False {
            }
            frame True {
              n786 = global read "全局 小时数据发送次数.vi" "小时数据发送次数"() -> (w1129:i32)
              n787 = Increment(x=w1129) -> (x+1=w1128:i32)
              n788 = global write "全局 小时数据发送次数.vi" "小时数据发送次数"(w1128) -> ()
            }
          }
        }
        frame "上传数据" {
          n789 = Index Array(array=w1134) -> (element=w1135:string)  [unwired: 1 in]
          n790 = case shown="\"原始时间\"" w1131 {
            tunnel: [w1145 w1147] -> w1136
            tunnel: w1135 -> [w1144 w1146]
            frame "精确到小时", Default {
              n791 = call "规范小时时间戳.vi"("字符串"=w1144) -> ("result string"=w1145:string)  [unwired: 10 in]
            }
            frame "原始时间" {
              n792 = call "日期字符串格式至时间格式转换(子VI).vi"("data[0]"=w1146) -> ("time stamp"=w1149:timestamp)  [unwired: 10 in]
              n793 = Seconds To Date/Time(time stamp (now)=w1149) -> (date time rec=w1148:T11)  [unwired: 1 in]
              n794 = Date/Time To Seconds(2:w1148) -> (0:w1150:timestamp)  [unwired: 1 in]
              n795 = Format Date/Time String(time format string (%c)="%Y%m%d%H%M%S" ("时间格式字符串(%c)"), seconds (now)=w1150) -> (date/time string=w1147:string)  [unwired: 1 in]
            }
          }
          n796 = call "关键参数组合 (子VI).vi"("table"="仪器参数", "因子编码"=w1133, "data"=w1134) -> ("字符串"=w1130:string)  [unwired: 8 in]
          n797 = Empty String/Path?(string/path=w1130) -> (empty?=w1143:bool)
          n798 = Format Into String(format string="DataTime=%s;%s" ("格式字符串"), w1136, w1130) -> (resulting string=w1138:string)  [unwired: 2 in, 1 out]
          n799 = String Length(string=w1138) -> (length=w1139:i32)
          n800 = Decrement(x=w1139) -> (x-1=w1140:i32)
          n801 = String Subset(string=w1138, length (rest)=w1140) -> (substring=w1137:string)  [unwired: 1 in]
          n802 = case shown="假" w1143 {
            tunnel: [w1152 ""] -> w1142
            tunnel: w1137 -> [w1152 _]
            frame False {
            }
            frame True {
            }
          }
        }
        frame "返回执行结果" {
        }
      }
    }
    frame "采配水仪器参数" {
      n803 = global read "全局1.vi" "枚举"() -> (w1158:enum16{"返回请求应答", "上传数据", "返回执行结果"})
      n804 = case shown="\"上传数据\"" w1158 {
        tunnel: ["QnRtn=1" w1183 "ExeRtn=1"] -> w1159
        tunnel: w1157 -> [_ w1171 _]
        tunnel: "w00000" -> [_ w1172 _]
        tunnel: w1156 -> [_ w1175 _]
        frame "返回请求应答", Default {
          n805 = global read "全局 数据数组大小.vi" "数据数组大小"() -> (w1162:i32)
          n806 = Equal To 0?(x=w1162) -> (x = 0?=w1161:bool)
          n807 = case shown="真" w1161 {
            frame False {
            }
            frame True {
              n808 = global read "全局 小时数据发送次数.vi" "小时数据发送次数"() -> (w1164:i32)
              n809 = Increment(x=w1164) -> (x+1=w1163:i32)
              n810 = global write "全局 小时数据发送次数.vi" "小时数据发送次数"(w1163) -> ()
            }
          }
        }
        frame "上传数据" {
          n811 = Index Array(array=w1171) -> (element=w1176:string)  [unwired: 1 in]
          n812 = case shown="\"原始时间\"" w1175 {
            tunnel: [w1186 w1188] -> w1177
            tunnel: w1176 -> [w1185 w1187]
            frame "精确到小时", Default {
              n813 = call "规范小时时间戳.vi"("字符串"=w1185) -> ("result string"=w1186:string)  [unwired: 10 in]
            }
            frame "原始时间" {
              n814 = call "日期字符串格式至时间格式转换(子VI).vi"("data[0]"=w1187) -> ("time stamp"=w1190:timestamp)  [unwired: 10 in]
              n815 = Seconds To Date/Time(time stamp (now)=w1190) -> (date time rec=w1189:T11)  [unwired: 1 in]
              n816 = Date/Time To Seconds(2:w1189) -> (0:w1191:timestamp)  [unwired: 1 in]
              n817 = Format Date/Time String(time format string (%c)="%Y%m%d%H%M%S" ("时间格式字符串(%c)"), seconds (now)=w1191) -> (date/time string=w1188:string)  [unwired: 1 in]
            }
          }
          n818 = Index Array(array=w1171, index #1=2 ("索引"), index #2=3 ("索引"), index #3=4 ("索引")) -> (element #1=w1167:string, element #2=w1166:string, element #3=w1165:string)
          n819 = Format Into String(format string="PolId=%s,i13111-Info=%s,i13112-Info=%s,i13113-Info=%s;", w1172, w1167, w1166, w1165) -> (resulting string=w1173:string)  [unwired: 2 in, 1 out]
          n820 = Empty String/Path?(string/path=w1173) -> (empty?=w1184:bool)
          n821 = Format Into String(format string="DataTime=%s;%s" ("格式字符串"), w1177, w1173) -> (resulting string=w1179:string)  [unwired: 2 in, 1 out]
          n822 = String Length(string=w1179) -> (length=w1180:i32)
          n823 = Decrement(x=w1180) -> (x-1=w1181:i32)
          n824 = String Subset(string=w1179, length (rest)=w1181) -> (substring=w1178:string)  [unwired: 1 in]
          n825 = case shown="假" w1184 {
            tunnel: [w1193 ""] -> w1183
            tunnel: w1178 -> [w1193 _]
            frame False {
            }
            frame True {
            }
          }
        }
        frame "返回执行结果" {
        }
      }
    }
    frame "3091校准信息" {
      n826 = case shown="\"CODMn\"" w1199 {
        selector: w1199 -> [w1203 _ _ _ _ _ _ _ _ _ _ _ _ _ _ _ _ _ _ _ _ _ _ _ _ _ _ _ _ _ _ _]
        tunnel: [w1203 w1206 w1210 w1214 w1218 w1222 w1226 w1230 w1234 w1238 w1242 w1246 w1250 w1254 w1258 w1262 w1266 w1270 w1274 w1278 w1282 w1286 w1290 w1294 w1298 w1302 w1306 w1310 w1314 w1318 w1322 w1326] -> w1198
        tunnel: [1.0 ("风向") w1204 w1208 w1212 w1216 w1220 w1224 w1228 w1232 w1236 w1240 w1244 w1248 w1252 w1256 w1260 w1264 w1268 w1272 w1276 w1280 w1284 w1288 w1292 w1296 w1300 w1304 w1308 w1312 w1316 w1320 w1324] -> _
        frame "假", Default {
        }
        frame "CODMn" {
          n827 = global read "断电保存全局.vi" "参数系数簇"() -> (w1205:T9)
          n828 = global read "断电保存全局.vi" "因子编码簇"() -> (w1207:T10)
          n829 = Unbundle By Name(w1205) -> ("CODMn"=w1204:dbl)
          n830 = Unbundle By Name(w1207) -> ("CODMn"=w1206:string)
        }
        frame "CODCr" {
          n831 = global read "断电保存全局.vi" "参数系数簇"() -> (w1209:T9)
          n832 = global read "断电保存全局.vi" "因子编码簇"() -> (w1211:T10)
          n833 = Unbundle By Name(w1209) -> ("CODCr"=w1208:dbl)
          n834 = Unbundle By Name(w1211) -> ("CODCr"=w1210:string)
        }
        frame "DO" {
          n835 = global read "断电保存全局.vi" "参数系数簇"() -> (w1213:T9)
          n836 = global read "断电保存全局.vi" "因子编码簇"() -> (w1215:T10)
          n837 = Unbundle By Name(w1213) -> ("DO"=w1212:dbl)
          n838 = Unbundle By Name(w1215) -> ("DO"=w1214:string)
        }
        frame "铜" {
          n839 = global read "断电保存全局.vi" "参数系数簇"() -> (w1217:T9)
          n840 = global read "断电保存全局.vi" "因子编码簇"() -> (w1219:T10)
          n841 = Unbundle By Name(w1217) -> ("铜"=w1216:dbl)
          n842 = Unbundle By Name(w1219) -> ("铜"=w1218:string)
        }
        frame "PH" {
          n843 = global read "断电保存全局.vi" "参数系数簇"() -> (w1221:T9)
          n844 = global read "断电保存全局.vi" "因子编码簇"() -> (w1223:T10)
          n845 = Unbundle By Name(w1221) -> ("PH"=w1220:dbl)
          n846 = Unbundle By Name(w1223) -> ("PH"=w1222:string)
        }
        frame "氨氮" {
          n847 = global read "断电保存全局.vi" "参数系数簇"() -> (w1225:T9)
          n848 = global read "断电保存全局.vi" "因子编码簇"() -> (w1227:T10)
          n849 = Unbundle By Name(w1225) -> ("氨氮"=w1224:dbl)
          n850 = Unbundle By Name(w1227) -> ("氨氮"=w1226:string)
        }
        frame "比电导率" {
          n851 = global read "断电保存全局.vi" "参数系数簇"() -> (w1229:T9)
          n852 = global read "断电保存全局.vi" "因子编码簇"() -> (w1231:T10)
          n853 = Unbundle By Name(w1229) -> ("比电导率"=w1228:dbl)
          n854 = Unbundle By Name(w1231) -> ("比电导率"=w1230:string)
        }
        frame "水温" {
          n855 = global read "断电保存全局.vi" "参数系数簇"() -> (w1233:T9)
          n856 = global read "断电保存全局.vi" "因子编码簇"() -> (w1235:T10)
          n857 = Unbundle By Name(w1233) -> ("水温"=w1232:dbl)
          n858 = Unbundle By Name(w1235) -> ("水温"=w1234:string)
        }
        frame "COD" {
          n859 = global read "断电保存全局.vi" "参数系数簇"() -> (w1237:T9)
          n860 = global read "断电保存全局.vi" "因子编码簇"() -> (w1239:T10)
          n861 = Unbundle By Name(w1237) -> ("COD"=w1236:dbl)
          n862 = Unbundle By Name(w1239) -> ("COD"=w1238:string)
        }
        frame "浊度" {
          n863 = global read "断电保存全局.vi" "参数系数簇"() -> (w1241:T9)
          n864 = global read "断电保存全局.vi" "因子编码簇"() -> (w1243:T10)
          n865 = Unbundle By Name(w1241) -> ("浊度"=w1240:dbl)
          n866 = Unbundle By Name(w1243) -> ("浊度"=w1242:string)
        }
        frame "总氮" {
          n867 = global read "断电保存全局.vi" "参数系数簇"() -> (w1245:T9)
          n868 = global read "断电保存全局.vi" "因子编码簇"() -> (w1247:T10)
          n869 = Unbundle By Name(w1245) -> ("总氮"=w1244:dbl)
          n870 = Unbundle By Name(w1247) -> ("总氮"=w1246:string)
        }
        frame "总磷" {
          n871 = global read "断电保存全局.vi" "参数系数簇"() -> (w1249:T9)
          n872 = global read "断电保存全局.vi" "因子编码簇"() -> (w1251:T10)
          n873 = Unbundle By Name(w1249) -> ("总磷"=w1248:dbl)
          n874 = Unbundle By Name(w1251) -> ("总磷"=w1250:string)
        }
        frame "叶绿素a" {
          n875 = global read "断电保存全局.vi" "参数系数簇"() -> (w1253:T9)
          n876 = global read "断电保存全局.vi" "因子编码簇"() -> (w1255:T10)
          n877 = Unbundle By Name(w1253) -> ("叶绿素a"=w1252:dbl)
          n878 = Unbundle By Name(w1255) -> ("叶绿素a"=w1254:string)
        }
        frame "藻密度" {
          n879 = global read "断电保存全局.vi" "参数系数簇"() -> (w1257:T9)
          n880 = global read "断电保存全局.vi" "因子编码簇"() -> (w1259:T10)
          n881 = Unbundle By Name(w1257) -> ("藻密度"=w1256:dbl)
          n882 = Unbundle By Name(w1259) -> ("藻密度"=w1258:string)
        }
        frame "水位" {
          n883 = global read "断电保存全局.vi" "参数系数簇"() -> (w1261:T9)
          n884 = global read "断电保存全局.vi" "因子编码簇"() -> (w1263:T10)
          n885 = Unbundle By Name(w1261) -> ("水位"=w1260:dbl)
          n886 = Unbundle By Name(w1263) -> ("水位"=w1262:string)
        }
        frame "流速" {
          n887 = global read "断电保存全局.vi" "参数系数簇"() -> (w1265:T9)
          n888 = global read "断电保存全局.vi" "因子编码簇"() -> (w1267:T10)
          n889 = Unbundle By Name(w1265) -> ("流速"=w1264:dbl)
          n890 = Unbundle By Name(w1267) -> ("流速"=w1266:string)
        }
        frame "瞬时流量" {
          n891 = global read "断电保存全局.vi" "参数系数簇"() -> (w1269:T9)
          n892 = global read "断电保存全局.vi" "因子编码簇"() -> (w1271:T10)
          n893 = Unbundle By Name(w1269) -> ("瞬时流量"=w1268:dbl)
          n894 = Unbundle By Name(w1271) -> ("瞬时流量"=w1270:string)
        }
        frame "累积流量" {
          n895 = global read "断电保存全局.vi" "参数系数簇"() -> (w1273:T9)
          n896 = global read "断电保存全局.vi" "因子编码簇"() -> (w1275:T10)
          n897 = Unbundle By Name(w1273) -> ("累积流量"=w1272:dbl)
          n898 = Unbundle By Name(w1275) -> ("累积流量"=w1274:string)
        }
        frame "亚硝酸盐" {
          n899 = global read "断电保存全局.vi" "参数系数簇"() -> (w1277:T9)
          n900 = global read "断电保存全局.vi" "因子编码簇"() -> (w1279:T10)
          n901 = Unbundle By Name(w1277) -> ("亚硝酸盐"=w1276:dbl)
          n902 = Unbundle By Name(w1279) -> ("亚硝酸盐"=w1278:string)
        }
        frame "硫化物" {
          n903 = global read "断电保存全局.vi" "参数系数簇"() -> (w1281:T9)
          n904 = global read "断电保存全局.vi" "因子编码簇"() -> (w1283:T10)
          n905 = Unbundle By Name(w1281) -> ("硫化物"=w1280:dbl)
          n906 = Unbundle By Name(w1283) -> ("硫化物"=w1282:string)
        }
        frame "ORP" {
          n907 = global read "断电保存全局.vi" "参数系数簇"() -> (w1285:T9)
          n908 = global read "断电保存全局.vi" "因子编码簇"() -> (w1287:T10)
          n909 = Unbundle By Name(w1285) -> ("ORP"=w1284:dbl)
          n910 = Unbundle By Name(w1287) -> ("ORP"=w1286:string)
        }
        frame "铅" {
          n911 = global read "断电保存全局.vi" "参数系数簇"() -> (w1289:T9)
          n912 = global read "断电保存全局.vi" "因子编码簇"() -> (w1291:T10)
          n913 = Unbundle By Name(w1289) -> ("铅"=w1288:dbl)
          n914 = Unbundle By Name(w1291) -> ("铅"=w1290:string)
        }
        frame "镉" {
          n915 = global read "断电保存全局.vi" "参数系数簇"() -> (w1293:T9)
          n916 = global read "断电保存全局.vi" "因子编码簇"() -> (w1295:T10)
          n917 = Unbundle By Name(w1293) -> ("镉"=w1292:dbl)
          n918 = Unbundle By Name(w1295) -> ("镉"=w1294:string)
        }
        frame "锌" {
          n919 = global read "断电保存全局.vi" "参数系数簇"() -> (w1297:T9)
          n920 = global read "断电保存全局.vi" "因子编码簇"() -> (w1299:T10)
          n921 = Unbundle By Name(w1297) -> ("锌"=w1296:dbl)
          n922 = Unbundle By Name(w1299) -> ("锌"=w1298:string)
        }
        frame "镍" {
          n923 = global read "断电保存全局.vi" "参数系数簇"() -> (w1301:T9)
          n924 = global read "断电保存全局.vi" "因子编码簇"() -> (w1303:T10)
          n925 = Unbundle By Name(w1301) -> ("镍"=w1300:dbl)
          n926 = Unbundle By Name(w1303) -> ("镍"=w1302:string)
        }
        frame "锰" {
          n927 = global read "断电保存全局.vi" "参数系数簇"() -> (w1305:T9)
          n928 = global read "断电保存全局.vi" "因子编码簇"() -> (w1307:T10)
          n929 = Unbundle By Name(w1305) -> ("锰"=w1304:dbl)
          n930 = Unbundle By Name(w1307) -> ("锰"=w1306:string)
        }
        frame "汞" {
          n931 = global read "断电保存全局.vi" "参数系数簇"() -> (w1309:T9)
          n932 = global read "断电保存全局.vi" "因子编码簇"() -> (w1311:T10)
          n933 = Unbundle By Name(w1309) -> ("汞"=w1308:dbl)
          n934 = Unbundle By Name(w1311) -> ("汞"=w1310:string)
        }
        frame "气温" {
          n935 = global read "断电保存全局.vi" "参数系数簇"() -> (w1313:T9)
          n936 = global read "断电保存全局.vi" "因子编码簇"() -> (w1315:T10)
          n937 = Unbundle By Name(w1313) -> ("气温"=w1312:dbl)
          n938 = Unbundle By Name(w1315) -> ("气温"=w1314:string)
        }
        frame "气压" {
          n939 = global read "断电保存全局.vi" "参数系数簇"() -> (w1317:T9)
          n940 = global read "断电保存全局.vi" "因子编码簇"() -> (w1319:T10)
          n941 = Unbundle By Name(w1317) -> ("气压"=w1316:dbl)
          n942 = Unbundle By Name(w1319) -> ("气压"=w1318:string)
        }
        frame "风速" {
          n943 = global read "断电保存全局.vi" "参数系数簇"() -> (w1321:T9)
          n944 = global read "断电保存全局.vi" "因子编码簇"() -> (w1323:T10)
          n945 = Unbundle By Name(w1321) -> ("风速"=w1320:dbl)
          n946 = Unbundle By Name(w1323) -> ("风速"=w1322:string)
        }
        frame "风向" {
          n947 = global read "断电保存全局.vi" "参数系数簇"() -> (w1325:T9)
          n948 = global read "断电保存全局.vi" "因子编码簇"() -> (w1327:T10)
          n949 = Unbundle By Name(w1325) -> ("风向"=w1324:dbl)
          n950 = Unbundle By Name(w1327) -> ("风向"=w1326:string)
        }
      }
      n951 = global read "全局1.vi" "枚举"() -> (w1200:enum16{"返回请求应答", "上传数据", "返回执行结果"})
      n952 = case shown="\"上传数据\"" w1200 {
        tunnel: ["QnRtn=1" w1344 "ExeRtn=1"] -> w1201
        tunnel: w1197 -> [_ w1334 _]
        tunnel: w1198 -> [_ w1333 _]
        tunnel: w1196 -> [_ w1336 _]
        frame "返回请求应答", Default {
          n953 = global read "全局 数据数组大小.vi" "数据数组大小"() -> (w1330:i32)
          n954 = Equal To 0?(x=w1330) -> (x = 0?=w1329:bool)
          n955 = case shown="真" w1329 {
            frame False {
            }
            frame True {
              n956 = global read "全局 小时数据发送次数.vi" "小时数据发送次数"() -> (w1332:i32)
              n957 = Increment(x=w1332) -> (x+1=w1331:i32)
              n958 = global write "全局 小时数据发送次数.vi" "小时数据发送次数"(w1331) -> ()
            }
          }
        }
        frame "上传数据" {
          n959 = call "校准信息组合 (子VI).vi"("因子编码"=w1333, "data"=w1334) -> ("字符串"=w1335:string)  [unwired: 9 in]
          n960 = Index Array(array=w1334) -> (element=w1337:string)  [unwired: 1 in]
          n961 = case shown="\"原始时间\"" w1336 {
            tunnel: [w1347 w1349] -> w1338
            tunnel: w1337 -> [w1346 w1348]
            frame "精确到小时", Default {
              n962 = call "规范小时时间戳.vi"("字符串"=w1346) -> ("result string"=w1347:string)  [unwired: 10 in]
            }
            frame "原始时间" {
              n963 = call "日期字符串格式至时间格式转换(子VI).vi"("data[0]"=w1348) -> ("time stamp"=w1351:timestamp)  [unwired: 10 in]
              n964 = Seconds To Date/Time(time stamp (now)=w1351) -> (date time rec=w1350:T11)  [unwired: 1 in]
              n965 = Date/Time To Seconds(2:w1350) -> (0:w1352:timestamp)  [unwired: 1 in]
              n966 = Format Date/Time String(time format string (%c)="%Y%m%d%H%M%S" ("时间格式字符串(%c)"), seconds (now)=w1352) -> (date/time string=w1349:string)  [unwired: 1 in]
            }
          }
          n967 = Empty String/Path?(string/path=w1335) -> (empty?=w1345:bool)
          n968 = Format Into String(format string="DataTime=%s;%s" ("格式字符串"), w1338, w1335) -> (resulting string=w1340:string)  [unwired: 2 in, 1 out]
          n969 = String Length(string=w1340) -> (length=w1341:i32)
          n970 = Decrement(x=w1341) -> (x-1=w1342:i32)
          n971 = String Subset(string=w1340, length (rest)=w1342) -> (substring=w1339:string)  [unwired: 1 in]
          n972 = case shown="假" w1345 {
            tunnel: [w1354 ""] -> w1344
            tunnel: w1339 -> [w1354 _]
            frame False {
            }
            frame True {
            }
          }
        }
        frame "返回执行结果" {
        }
      }
    }
    frame "3090仪器参数" {
      n973 = global read "全局 小时数据发送次数.vi" "小时数据发送次数"() -> (w1359:i32)
      n974 = Index Array(array=w1361, index (row)=w1359) -> (element=w1358:string[])  [unwired: 1 in]
      n975 = global read "全局1.vi" "枚举"() -> (w1360:enum16{"返回请求应答", "上传数据", "返回执行结果"})
      n976 = case shown="\"上传数据\"" w1360 {
        tunnel: ["QnRtn=1" w1379 "ExeRtn=1"] -> w1362
        tunnel: w1358 -> [_ w1376 _]
        tunnel: w1357 -> [_ w1369 _]
        frame "返回请求应答", Default {
          n977 = global read "全局 数据数组大小.vi" "数据数组大小"() -> (w1365:i32)
          n978 = Equal To 0?(x=w1365) -> (x = 0?=w1364:bool)
          n979 = case shown="真" w1364 {
            frame False {
            }
            frame True {
              n980 = global read "全局 小时数据发送次数.vi" "小时数据发送次数"() -> (w1367:i32)
              n981 = Increment(x=w1367) -> (x+1=w1366:i32)
              n982 = global write "全局 小时数据发送次数.vi" "小时数据发送次数"(w1366) -> ()
            }
          }
        }
        frame "上传数据" {
          n983 = Index Array(array=w1376) -> (element=w1375:string)  [unwired: 1 in]
          n984 = call "数据发送组合-20200825 (子VI).vi"("枚举"=T6."3090仪器参数", "插值后的数组元素"=w1369) -> ("字符串"=w1368:string)  [unwired: 9 in]
          n985 = call "规范时间戳.vi"("字符串"=w1375) -> ("result string"=w1377:string)  [unwired: 10 in]
          n986 = Format Into String(format string="DataTime=%s;%s" ("格式字符串"), w1377, w1368) -> (resulting string=w1372:string)  [unwired: 2 in, 1 out]
          n987 = String Length(string=w1372) -> (length=w1373:i32)
          n988 = Decrement(x=w1373) -> (x-1=w1374:i32)
          n989 = String Subset(string=w1372, length (rest)=w1374) -> (substring=w1371:string)  [unwired: 1 in]
          n990 = Empty String/Path?(string/path=w1371) -> (empty?=w1380:bool)
          n991 = case shown="假" w1380 {
            tunnel: [w1383 ""] -> w1379
            tunnel: w1371 -> [w1383 _]
            frame False {
              n992 = global read "全局 小时数据发送次数.vi" "小时数据发送次数"() -> (w1382:i32)
              n993 = Increment(x=w1382) -> (x+1=w1381:i32)
              n994 = global write "全局 小时数据发送次数.vi" "小时数据发送次数"(w1381) -> ()
            }
            frame True {
              n995 = global read "全局 小时数据发送次数.vi" "小时数据发送次数"() -> (w1385:i32)
              n996 = Increment(x=w1385) -> (x+1=w1384:i32)
              n997 = global write "全局 小时数据发送次数.vi" "小时数据发送次数"(w1384) -> ()
            }
          }
        }
        frame "返回执行结果" {
        }
      }
    }
    frame "提取仪器参数" {
      n998 = global read "全局1.vi" "枚举"() -> (w1389:enum16{"返回请求应答", "上传数据", "返回执行结果"})
      n999 = case shown="\"上传数据\"" w1389 {
        tunnel: ["QnRtn=1" w1399 "ExeRtn=1"] -> w1390
        tunnel: w1388 -> [_ w1397 _]
        frame "返回请求应答", Default {
          n1000 = global read "全局 数据数组大小.vi" "数据数组大小"() -> (w1393:i32)
          n1001 = Equal To 0?(x=w1393) -> (x = 0?=w1392:bool)
          n1002 = case shown="假" w1392 {
            frame False {
            }
            frame True {
              n1003 = global read "全局 小时数据发送次数.vi" "小时数据发送次数"() -> (w1395:i32)
              n1004 = Increment(x=w1395) -> (x+1=w1394:i32)
              n1005 = global write "全局 小时数据发送次数.vi" "小时数据发送次数"(w1394) -> ()
            }
          }
        }
        frame "上传数据" {
          n1006 = call "数据发送组合-20200825 (子VI).vi"("枚举"=T6."提取仪器参数", "插值后的数组元素"=w1397) -> ("字符串"=w1396:string)  [unwired: 9 in]
          n1007 = Empty String/Path?(string/path=w1396) -> (empty?=w1400:bool)
          n1008 = case shown="假" w1400 {
            tunnel: [w1403 ""] -> w1399
            tunnel: w1396 -> [w1403 _]
            frame False {
              n1009 = global read "全局 小时数据发送次数.vi" "小时数据发送次数"() -> (w1402:i32)
              n1010 = Increment(x=w1402) -> (x+1=w1401:i32)
              n1011 = global write "全局 小时数据发送次数.vi" "小时数据发送次数"(w1401) -> ()
            }
            frame True {
              n1012 = global read "全局 小时数据发送次数.vi" "小时数据发送次数"() -> (w1405:i32)
              n1013 = Increment(x=w1405) -> (x+1=w1404:i32)
              n1014 = global write "全局 小时数据发送次数.vi" "小时数据发送次数"(w1404) -> ()
            }
          }
        }
        frame "返回执行结果" {
        }
      }
    }
    frame "报警信息" {
      n1015 = global read "全局 小时数据发送次数.vi" "小时数据发送次数"() -> (w1410:i32)
      n1016 = Index Array(array=w1412, index (row)=w1410) -> (element=w1409:string[])  [unwired: 1 in]
      n1017 = global read "全局1.vi" "枚举"() -> (w1411:enum16{"返回请求应答", "上传数据", "返回执行结果"})
      n1018 = case shown="\"上传数据\"" w1411 {
        tunnel: ["QnRtn=1" w1425 "ExeRtn=1"] -> w1413
        tunnel: w1409 -> [_ _ _]
        tunnel: w1408 -> [_ w1420 _]
        frame "返回请求应答", Default {
          n1019 = global read "全局 数据数组大小.vi" "数据数组大小"() -> (w1416:i32)
          n1020 = Equal To 0?(x=w1416) -> (x = 0?=w1415:bool)
          n1021 = case shown="真" w1415 {
            frame False {
            }
            frame True {
              n1022 = global read "全局 小时数据发送次数.vi" "小时数据发送次数"() -> (w1418:i32)
              n1023 = Increment(x=w1418) -> (x+1=w1417:i32)
              n1024 = global write "全局 小时数据发送次数.vi" "小时数据发送次数"(w1417) -> ()
            }
          }
        }
        frame "上传数据" {
          n1025 = call "数据发送组合-20200825 (子VI).vi"("枚举"=T6."报警信息", "插值后的数组元素"=w1420) -> ("字符串"=w1419:string)  [unwired: 9 in]
          n1026 = Empty String/Path?(string/path=w1419) -> (empty?=w1426:bool)
          n1027 = String Length(string=w1419) -> (length=w1424:i32)
          n1028 = Decrement(x=w1424) -> (x-1=w1423:i32)
          n1029 = String Subset(string=w1419, length (rest)=w1423) -> (substring=w1422:string)  [unwired: 1 in]
          n1030 = case shown="假" w1426 {
            tunnel: [w1429 ""] -> w1425
            tunnel: w1422 -> [w1429 _]
            frame False {
              n1031 = global read "全局 小时数据发送次数.vi" "小时数据发送次数"() -> (w1428:i32)
              n1032 = Increment(x=w1428) -> (x+1=w1427:i32)
              n1033 = global write "全局 小时数据发送次数.vi" "小时数据发送次数"(w1427) -> ()
            }
            frame True {
              n1034 = global read "全局 小时数据发送次数.vi" "小时数据发送次数"() -> (w1431:i32)
              n1035 = Increment(x=w1431) -> (x+1=w1430:i32)
              n1036 = global write "全局 小时数据发送次数.vi" "小时数据发送次数"(w1430) -> ()
            }
          }
        }
        frame "返回执行结果" {
        }
      }
    }
    frame "系统状态" {
      # ",i12002-Info=0,i12003-Info=100,i12031-Info=0"
      # "DataTime=20100301145000;PolId=w01018,i12001-Info=1,i12003-Info=100"
      # "100  当前模式\n101  CODMn状态  （0待机，1运行）\n102  氨氮状态\n103  总磷状态\n104  总氮状态\n105  CODCr状态\n106  运行周期"
      n1037 = global read "全局 小时数据发送次数.vi" "小时数据发送次数"() -> (w1438:i32)
      n1038 = Build Array("w00000", "w01019", "w21003", "w21011", "w21001", "w01018") -> (w1441:string[])
      n1039 = global read "全局1.vi" "register values"() -> (w1439:u16[])
      n1040 = Index Array(array=w1439, index=w1438) -> (element=w1437:u16)
      n1041 = Index Array(array=w1441, index=w1438) -> (element=w1440:string)
      n1042 = case shown="1, 默认" w1438 {
        tunnel: w1440 -> [w1456 w1461]
        tunnel: w1437 -> [w1457 _]
        tunnel: [w1454 w1460] -> w1436
        frame 1, Default {
          n1043 = Number To Decimal String(number=w1457) -> (decimal integer string=w1458:string)  [unwired: 1 in]
          n1044 = Format Into String(w1458) -> (resulting string=w1455:string)  [unwired: 3 in, 1 out]
          n1045 = Format Into String(format string="PolId=%s,i12001-Info=%s,i12002-Info=0;" ("格式字符串"), w1456, w1455) -> (resulting string=w1454:string)  [unwired: 2 in, 1 out]
        }
        frame 0 {
          n1046 = Format Into String(format string="PolId=%s,i22001-Info=0,i22002-Info=1,i22003-Info=0;" ("格式字符串"), w1461) -> (resulting string=w1460:string)  [unwired: 2 in, 1 out]
        }
      }
      n1047 = Get Date/Time In Seconds() -> (seconds since 1Jan1904=w1451:timestamp)
      n1048 = Format Date/Time String(time format string (%c)="%Y%m%d%H%M%S" ("时间格式字符串(%c)"), seconds (now)=w1451) -> (date/time string=w1450:string)  [unwired: 1 in]
      n1049 = Format Into String(format string="DataTime=%s;%s" ("格式字符串"), w1450, w1436) -> (resulting string=w1447:string)  [unwired: 2 in, 1 out]
      n1050 = String Length(string=w1447) -> (length=w1449:i32)
      n1051 = Decrement(x=w1449) -> (x-1=w1448:i32)
      n1052 = String Subset(string=w1447, length (rest)=w1448) -> (substring=w1446:string)  [unwired: 1 in]
    }
    frame "运行模式" {
      # "DataTime=20100301145000;PolId=w01018,i12001-Info=1,i12003-Info=0"
      # "100  当前模式\n101  CODMn状态  （0待机，1运行）\n102  氨氮状态\n103  总磷状态\n104  总氮状态\n105  CODCr状态\n106  运行周期"
      n1053 = Get Date/Time In Seconds() -> (seconds since 1Jan1904=w1470:timestamp)
      n1054 = Format Date/Time String(time format string (%c)="%Y%m%d%H%M%S" ("时间格式字符串(%c)"), seconds (now)=w1470) -> (date/time string=w1467:string)  [unwired: 1 in]
      n1055 = global read "全局1.vi" "register values"() -> (w1472:u16[])
      n1056 = Index Array(array=w1472, index=0 ("索引")) -> (element=w1464:u16)
      n1057 = Number To Decimal String(number=w1464) -> (decimal integer string=w1466:string)  [unwired: 1 in]
      n1058 = Format Into String(format string="RunMode=%s;" ("格式字符串"), w1466) -> (resulting string=w1463:string)  [unwired: 2 in, 1 out]
      n1059 = Format Into String(format string="DataTime=%s;%s" ("格式字符串"), w1467, w1463) -> (resulting string=w1469:string)  [unwired: 2 in, 1 out]
    }
    frame "测量周期" {
      n1060 = global read "全局1.vi" "register values"() -> (w1483:u16[])
      n1061 = Index Array(array=w1483, index=6 ("索引")) -> (element=w1475:u16)
      n1062 = Get Date/Time In Seconds() -> (seconds since 1Jan1904=w1481:timestamp)
      n1063 = Format Date/Time String(time format string (%c)="%Y%m%d%H%M%S" ("时间格式字符串(%c)"), seconds (now)=w1481) -> (date/time string=w1478:string)  [unwired: 1 in]
      n1064 = Number To Decimal String(number=w1475) -> (decimal integer string=w1476:string)  [unwired: 1 in]
      n1065 = Format Into String(format string="RunInterval=%s;" ("格式字符串"), w1476) -> (resulting string=w1474:string)  [unwired: 2 in, 1 out]
      n1066 = Format Into String(format string="DataTime=%s;%s" ("格式字符串"), w1478, w1474) -> (resulting string=w1480:string)  [unwired: 2 in, 1 out]
    }
    frame "各参数测量周期" {
      # "QN=20101108135153914;ST=21;CN=2084;PW=123456;MN=A110000_0001;Flag=9;CP=&&DataTime=20100301145000;PolId=w01018,RunInterval=4;PolId=w01019,RunInterval=4;...&&"
      n1067 = global read "全局1.vi" "读取各参数测量周期的值"() -> (w1486:u16[])
      n1068 = Get Date/Time In Seconds() -> (seconds since 1Jan1904=w1489:timestamp)
      n1069 = call "2084上传各参数测量周期.vi"("读取各参数测量周期的值"=w1486) -> ("字符串"=w1485:string)  [unwired: 10 in]
      n1070 = Format Date/Time String(time format string (%c)="%Y%m%d%H%M%S" ("时间格式字符串(%c)"), seconds (now)=w1489) -> (date/time string=w1487:string)  [unwired: 1 in]
      n1071 = Format Into String(format string="DataTime=%s;%s" ("格式字符串"), w1487, w1485) -> (resulting string=w1488:string)  [unwired: 2 in, 1 out]
    }
    frame "超标留样" {
      # "DataTime=20100301145000;PolId=w01018,i12001-Info=1,i12003-Info=0"
      # "100  当前模式\n101  CODMn状态  （0待机，1运行）\n102  氨氮状态\n103  总磷状态\n104  总氮状态\n105  CODCr状态\n106  运行周期"
      n1072 = global read "全局1.vi" "register values"() -> (w1501:u16[])
      n1073 = Get Date/Time In Seconds() -> (seconds since 1Jan1904=w1499:timestamp)
      n1074 = Format Date/Time String(time format string (%c)="%Y%m%d%H%M%S" ("时间格式字符串(%c)"), seconds (now)=w1499) -> (date/time string=w1496:string)  [unwired: 1 in]
      n1075 = Index Array(array=w1501, index=7 ("索引")) -> (element=w1493:u16)
      n1076 = Number To Decimal String(number=w1493) -> (decimal integer string=w1494:string)  [unwired: 1 in]
      n1077 = Format Into String(format string="VaseNo=%s;" ("格式字符串"), w1494) -> (resulting string=w1492:string)  [unwired: 2 in, 1 out]
      n1078 = Format Into String(format string="DataTime=%s;%s" ("格式字符串"), w1496, w1492) -> (resulting string=w1498:string)  [unwired: 2 in, 1 out]
    }
    frame "3201告警信息" {
      n1079 = global read "全局 小时数据发送次数.vi" "小时数据发送次数"() -> (w1503:i32)
      n1080 = Get Date/Time In Seconds() -> (seconds since 1Jan1904=w1509:timestamp)
      n1081 = Format Date/Time String(time format string (%c)="%Y%m%d%H%M%S" ("时间格式字符串(%c)"), seconds (now)=w1509) -> (date/time string=w1507:string)  [unwired: 1 in]
      n1082 = Number To Decimal String(number=w1503) -> (decimal integer string=w1504:string)  [unwired: 1 in]
      n1083 = Format Into String(format string="SystemAlarm=%s" ("格式字符串"), w1504) -> (resulting string=w1505:string)  [unwired: 2 in, 1 out]
      n1084 = Format Into String(format string="DataTime=%s;%s" ("格式字符串"), w1507, w1505) -> (resulting string=w1508:string)  [unwired: 2 in, 1 out]
    }
  }
  n1085 = case shown="假" w24 {
    tunnel: [w1513 w1517] -> w26
    frame False {
      n1086 = global read "全局1.vi" "枚举"() -> (w1512:enum16{"返回请求应答", "上传数据", "返回执行结果"})
      n1087 = case shown="\"上传数据\"" w1512 {
        tunnel: ["91" ("CN") w1515 "91" ("CN")] -> w1513
        frame "返回请求应答", Default {
        }
        frame "上传数据" {
          n1088 = global read "全局1.vi" "系统编码ST"() -> (w1515:string)
        }
        frame "返回执行结果" {
        }
      }
    }
    frame True {
      n1089 = global read "全局 反控命令枚举.vi" "反控命令枚举"() -> (w1518:enum16{"返回请求应答", "返回执行结果"})
      n1090 = case shown="\"返回执行结果\"" w1518 {
        tunnel: ["91" "91"] -> w1517
        frame "返回请求应答", Default {
        }
        frame "返回执行结果" {
        }
      }
    }
  }
  n1091 = case shown="\"获取仪器软件版本号\"" "table输入" {
    tunnel: ["9015" ("ST") w1531 w1539 w1547 w1554 w1561 w1569 w1577 w1585 w1593 w1602 w1617 w1629 w1637 w1645 w1654 w1663 w1680 w1688 w1696 w1704 w1712 w1720 w1731 w1743 w1755 w1767 w1779 w1787 "3020" ("ST") "3042" ("ST") "3056" ("ST") "2084" ("ST") "3015" ("ST") "3201" ("ST")] -> w29
    tunnel: ["9" ("ST") "9" ("ST") "9" ("ST") "8" ("ST") "8" ("ST") "9" ("ST") "9" ("ST") "9" ("ST") "8" ("ST") "8" ("ST") "9" ("ST") "9" ("ST") "11" ("ST") "9" ("ST") "9" ("ST") w1657 "9" ("ST") "9" ("ST") "9" ("ST") "9" ("ST") "9" ("ST") "9" ("ST") "9" ("ST") "9" ("ST") "9" ("ST") "9" ("ST") "9" ("ST") "9" ("ST") "9" ("ST") "9" ("ST") "9" ("ST") "9" ("ST") "9" ("ST") "9" ("ST") "9" ("ST")] -> w28
    tunnel: w19 -> [_ w1529 w1537 w1548 w1555 w1562 w1570 w1578 w1586 w1594 w1603 w1619 w1631 w1639 w1647 w1656 w1666 w1682 w1690 w1698 w1706 w1714 w1722 w1733 w1745 w1757 w1769 w1781 w1789 w1795 w1799 w1803 w1807 w1811 w1815]
    tunnel: [_ w1529 w1537 w1548 w1555 w1562 w1570 w1578 w1586 w1594 w1603 w1619 w1631 w1639 w1647 w1656 w1666 w1682 w1690 w1698 w1706 w1714 w1722 w1733 w1745 w1757 w1769 w1781 w1789 w1795 w1799 w1803 w1807 w1811 w1815] -> w8
    tunnel: [w1521 w1528 w1536 w1544 w1552 w1559 w1567 w1575 w1583 w1591 w1599 w1616 w1628 w1636 w1644 w1653 w1665 w1678 w1686 w1694 w1702 w1710 w1718 w1726 w1738 w1750 w1762 w1774 w1786 w1794 w1798 w1802 w1806 w1810 w1814] -> w20
    tunnel: [_ _ _ _ _ _ _ _ _ _ _ _ w1626 _ _ _ _ _ _ _ _ _ _ _ _ _ _ _ _ _ _ _ _ _ _] -> w6
    tunnel: [_ _ _ _ _ _ _ _ _ _ _ _ w1624 _ _ _ _ _ _ _ _ _ _ _ _ _ _ _ _ _ _ _ _ _ _] -> w5
    frame "心跳包", Default {
      # "心跳包"
      n1092 = Get Date/Time In Seconds() -> (seconds since 1Jan1904=w1524:timestamp)
      n1093 = Format Date/Time String(time format string (%c)="%Y%m%d%H%M%S%3u" ("时间格式字符串(%c)"), seconds (now)=w1524) -> (date/time string=w1523:string)  [unwired: 1 in]
      n1094 = Search and Replace String(input string=w1523, search string="." ("搜索字符串")) -> (result string=w1521:string)  [unwired: 6 in, 3 out]
    }
    frame "提取数采仪时间" {
      n1095 = global read "全局1.vi" "枚举"() -> (w1532:enum16{"返回请求应答", "上传数据", "返回执行结果"})
      n1096 = case shown="\"返回执行结果\"" w1532 {
        tunnel: ["9011" ("CN") "1014" ("CN") "9012" ("CN")] -> w1531
        frame "返回请求应答", Default {
        }
        frame "上传数据" {
        }
        frame "返回执行结果" {
        }
      }
      n1097 = local read "QN"() -> (w1528:string)
    }
    frame "提取实时数据间隔" {
      n1098 = global read "全局1.vi" "枚举"() -> (w1540:enum16{"返回请求应答", "上传数据", "返回执行结果"})
      n1099 = case shown="\"上传数据\"" w1540 {
        tunnel: ["9011" ("CN") "1061" ("CN") "9012" ("CN")] -> w1539
        frame "返回请求应答", Default {
        }
        frame "上传数据" {
        }
        frame "返回执行结果" {
        }
      }
      n1100 = local read "QN"() -> (w1536:string)
    }
    frame "反控命令" {
      n1101 = global read "全局 反控命令枚举.vi" "反控命令枚举"() -> (w1545:enum16{"返回请求应答", "返回执行结果"})
      n1102 = case shown="\"返回请求应答\", 默认" w1545 {
        tunnel: ["9011" ("CN") "9012" ("CN")] -> w1547
        frame "返回请求应答", Default {
        }
        frame "返回执行结果" {
        }
      }
      n1103 = local read "QN"() -> (w1544:string)
    }
    frame "超标留样返回" {
      n1104 = global read "全局1.vi" "枚举"() -> (w1551:enum16{"返回请求应答", "上传数据", "返回执行结果"})
      n1105 = case shown="\"上传数据\"" w1551 {
        tunnel: ["9011" ("CN") "3015" ("CN") "9012" ("CN")] -> w1554
        frame "返回请求应答", Default {
        }
        frame "上传数据" {
        }
        frame "返回执行结果" {
        }
      }
      n1106 = local read "QN"() -> (w1552:string)
    }
    frame "提取经纬度环境信息" {
      n1107 = global read "全局1.vi" "枚举"() -> (w1563:enum16{"返回请求应答", "上传数据", "返回执行结果"})
      n1108 = case shown="\"上传数据\"" w1563 {
        tunnel: ["9011" ("CN") "3041" ("CN") "9012" ("CN")] -> w1561
        frame "返回请求应答", Default {
        }
        frame "上传数据" {
        }
        frame "返回执行结果" {
        }
      }
      n1109 = local read "QN"() -> (w1559:string)
    }
    frame "提取现场系统信息" {
      n1110 = global read "全局1.vi" "枚举"() -> (w1571:enum16{"返回请求应答", "上传数据", "返回执行结果"})
      n1111 = case shown="\"上传数据\"" w1571 {
        tunnel: ["9011" ("CN") "3040" ("CN") "9012" ("CN")] -> w1569
        frame "返回请求应答", Default {
        }
        frame "上传数据" {
        }
        frame "返回执行结果" {
        }
      }
      n1112 = local read "QN"() -> (w1567:string)
    }
    frame "提取监测仪表时间" {
      n1113 = global read "全局1.vi" "枚举"() -> (w1579:enum16{"返回请求应答", "上传数据", "返回执行结果"})
      n1114 = case shown="\"上传数据\"" w1579 {
        tunnel: ["9011" ("CN") "1011" ("CN") "9012" ("CN")] -> w1577
        frame "返回请求应答", Default {
        }
        frame "上传数据" {
        }
        frame "返回执行结果" {
        }
      }
      n1115 = local read "QN"() -> (w1575:string)
    }
    frame "获取软件版本号" {
      n1116 = global read "全局1.vi" "枚举"() -> (w1587:enum16{"返回请求应答", "上传数据", "返回执行结果"})
      n1117 = case shown="\"返回执行结果\"" w1587 {
        tunnel: ["9011" ("CN") "3100" ("CN") "9012" ("CN")] -> w1585
        frame "返回请求应答", Default {
        }
        frame "上传数据" {
        }
        frame "返回执行结果" {
        }
      }
      n1118 = local read "QN"() -> (w1583:string)
    }
    frame "获取仪器软件版本号" {
      n1119 = global read "全局1.vi" "枚举"() -> (w1595:enum16{"返回请求应答", "上传数据", "返回执行结果"})
      n1120 = case shown="\"上传数据\"" w1595 {
        tunnel: ["9011" ("CN") "3102" ("CN") "9012" ("CN")] -> w1593
        frame "返回请求应答", Default {
        }
        frame "上传数据" {
        }
        frame "返回执行结果" {
        }
      }
      n1121 = local read "QN"() -> (w1591:string)
    }
    frame "实时数据" {
      n1122 = global read "全局1.vi" "枚举"() -> (w1601:enum16{"返回请求应答", "上传数据", "返回执行结果"})
      n1123 = case shown="\"上传数据\"" w1601 {
        tunnel: ["9011" ("CN") w1606 "9012" ("CN")] -> w1602
        frame "返回请求应答", Default {
        }
        frame "上传数据" {
          n1124 = global read "全局 实时数据参数.vi" "实时数据参数"() -> (w1605:string)
          n1125 = case shown="\"平行样测试\"" w1605 {
            tunnel: ["2011" ("CN") "2064" ("CN") "2082" ("CN") "2063" ("CN") "2062" ("CN") "2065" ("CN") "2066" ("CN") "fff" ("CN")] -> w1606
            frame "水样测试", Default {
            }
            frame "平行样测试" {
            }
            frame "集成干预测试" {
            }
            frame "加标回收测试" {
            }
            frame "核查数据" {
            }
            frame "空白测试" {
            }
            frame "跨度核查" {
            }
            frame "" {
            }
          }
        }
        frame "返回执行结果" {
        }
      }
      n1126 = local read "QN"() -> (w1599:string)
    }
    frame "小时数据" {
      # "监测小时数据"
      n1127 = global read "全局1.vi" "枚举"() -> (w1618:enum16{"返回请求应答", "上传数据", "返回执行结果"})
      n1128 = case shown="\"上传数据\"" w1618 {
        tunnel: ["9011" ("CN") "2061" ("CN") "9012" ("CN")] -> w1617
        frame "返回请求应答", Default {
        }
        frame "上传数据" {
        }
        frame "返回执行结果" {
        }
      }
      n1129 = local read "QN"() -> (w1616:string)
    }
    frame "剖面数据" {
      n1130 = global read "全局1.vi" "枚举"() -> (w1630:enum16{"返回请求应答", "上传数据", "返回执行结果"})
      n1131 = case shown="\"上传数据\"" w1630 {
        tunnel: ["9011" ("CN") "2083" ("CN") "9012" ("CN")] -> w1629
        frame "返回请求应答", Default {
        }
        frame "上传数据" {
        }
        frame "返回执行结果" {
        }
      }
      n1132 = global read "全局 数据数组大小.vi" "当前包号"() -> (w1625:i32)
      n1133 = global read "全局 数据数组大小.vi" "总包数"() -> (w1627:i32)
      n1134 = Number To Decimal String(number=w1627) -> (decimal integer string=w1626:string)  [unwired: 1 in]
      n1135 = Number To Decimal String(number=w1625) -> (decimal integer string=w1624:string)  [unwired: 1 in]
      n1136 = local read "QN"() -> (w1628:string)
    }
    frame "剖面多参数H" {
      # "监测小时数据"
      n1137 = global read "全局1.vi" "枚举"() -> (w1638:enum16{"返回请求应答", "上传数据", "返回执行结果"})
      n1138 = case shown="\"上传数据\"" w1638 {
        tunnel: ["9011" ("CN") "2061" ("CN") "9012" ("CN")] -> w1637
        frame "返回请求应答", Default {
        }
        frame "上传数据" {
        }
        frame "返回执行结果" {
        }
      }
      n1139 = local read "QN"() -> (w1636:string)
    }
    frame "剖面多参数S" {
      # "监测小时数据"
      n1140 = global read "全局1.vi" "枚举"() -> (w1646:enum16{"返回请求应答", "上传数据", "返回执行结果"})
      n1141 = case shown="\"上传数据\"" w1646 {
        tunnel: ["9011" ("CN") "2011" ("CN") "9012" ("CN")] -> w1645
        frame "返回请求应答", Default {
        }
        frame "上传数据" {
        }
        frame "返回执行结果" {
        }
      }
      n1142 = local read "QN"() -> (w1644:string)
    }
    frame "提取小时数据" {
      # "监测小时数据"
      n1143 = global read "全局1.vi" "枚举"() -> (w1655:enum16{"返回请求应答", "上传数据", "返回执行结果"})
      n1144 = global read "断电保存全局.vi" "数据组合发送"() -> (w1652:bool)
      n1145 = case shown="\"上传数据\"" w1655 {
        tunnel: ["9011" ("CN") "2061" ("CN") "9012" ("CN")] -> w1654
        frame "返回请求应答", Default {
        }
        frame "上传数据" {
        }
        frame "返回执行结果" {
        }
      }
      n1146 = case shown="假" w1652 {
        tunnel: ["9" ("ST") "9" ("ST")] -> w1657
        frame False {
        }
        frame True {
        }
      }
      n1147 = local read "QN"() -> (w1653:string)
    }
    frame "提取实时数据" {
      # "提取实时数据"
      n1148 = global read "全局1.vi" "枚举"() -> (w1664:enum16{"返回请求应答", "上传数据", "返回执行结果"})
      n1149 = case shown="\"上传数据\"" w1664 {
        tunnel: ["9011" ("CN") w1670 "9012" ("CN")] -> w1663
        frame "返回请求应答", Default {
        }
        frame "上传数据" {
          n1150 = global read "全局 实时数据参数.vi" "实时数据参数"() -> (w1669:string)
          n1151 = case shown="\"平行样测试\"" w1669 {
            tunnel: ["2011" ("CN") "2064" ("CN") "2063" ("CN") "2065" ("CN") "2066" ("CN") "fff" ("CN")] -> w1670
            frame "水样测试", Default {
            }
            frame "平行样测试" {
            }
            frame "加标回收测试" {
            }
            frame "空白测试" {
            }
            frame "跨度核查" {
            }
            frame "" {
            }
          }
        }
        frame "返回执行结果" {
        }
      }
      n1152 = local read "QN"() -> (w1665:string)
    }
    frame "跨度核查" {
      # "跨度核查"
      n1153 = global read "全局1.vi" "枚举"() -> (w1681:enum16{"返回请求应答", "上传数据", "返回执行结果"})
      n1154 = case shown="\"上传数据\"" w1681 {
        tunnel: ["9011" ("CN") "2066" ("ST") "9012" ("CN")] -> w1680
        frame "返回请求应答", Default {
        }
        frame "上传数据" {
        }
        frame "返回执行结果" {
        }
      }
      n1155 = local read "QN"() -> (w1678:string)
    }
    frame "提取加标回收" {
      # "提取加标回收"
      n1156 = global read "全局1.vi" "枚举"() -> (w1689:enum16{"返回请求应答", "上传数据", "返回执行结果"})
      n1157 = case shown="\"上传数据\"" w1689 {
        tunnel: ["9011" ("CN") "2063" ("ST") "9012" ("CN")] -> w1688
        frame "返回请求应答", Default {
        }
        frame "上传数据" {
        }
        frame "返回执行结果" {
        }
      }
      n1158 = local read "QN"() -> (w1686:string)
    }
    frame "提取平行样" {
      # "提取平行样"
      n1159 = global read "全局1.vi" "枚举"() -> (w1697:enum16{"返回请求应答", "上传数据", "返回执行结果"})
      n1160 = case shown="\"上传数据\"" w1697 {
        tunnel: ["9011" ("CN") "2064" ("ST") "9012" ("CN")] -> w1696
        frame "返回请求应答", Default {
        }
        frame "上传数据" {
        }
        frame "返回执行结果" {
        }
      }
      n1161 = local read "QN"() -> (w1694:string)
    }
    frame "空白测试", "零点核查" {
      # "零点核查"
      n1162 = global read "全局1.vi" "枚举"() -> (w1705:enum16{"返回请求应答", "上传数据", "返回执行结果"})
      n1163 = case shown="\"上传数据\"" w1705 {
        tunnel: ["9011" ("CN") "2065" ("ST") "9012" ("CN")] -> w1704
        frame "返回请求应答", Default {
        }
        frame "上传数据" {
        }
        frame "返回执行结果" {
        }
      }
      n1164 = local read "QN"() -> (w1702:string)
    }
    frame "核查数据" {
      # "核查数据"
      n1165 = global read "全局1.vi" "枚举"() -> (w1713:enum16{"返回请求应答", "上传数据", "返回执行结果"})
      n1166 = case shown="\"上传数据\"" w1713 {
        tunnel: ["9011" ("CN") "2062" ("ST") "9012" ("CN")] -> w1712
        frame "返回请求应答", Default {
        }
        frame "上传数据" {
        }
        frame "返回执行结果" {
        }
      }
      n1167 = local read "QN"() -> (w1710:string)
    }
    frame "提取集成干预" {
      # "核查数据"
      n1168 = global read "全局1.vi" "枚举"() -> (w1721:enum16{"返回请求应答", "上传数据", "返回执行结果"})
      n1169 = case shown="\"上传数据\"" w1721 {
        tunnel: ["9011" ("CN") "2082" ("ST") "9012" ("CN")] -> w1720
        frame "返回请求应答", Default {
        }
        frame "上传数据" {
        }
        frame "返回执行结果" {
        }
      }
      n1170 = local read "QN"() -> (w1718:string)
    }
    frame "报警信息", "采配水仪器参数", "操作日志", "仪器参数" {
      n1171 = global read "全局1.vi" "枚举"() -> (w1732:enum16{"返回请求应答", "上传数据", "返回执行结果"})
      n1172 = case shown="\"上传数据\"" w1732 {
        tunnel: ["9011" ("CN") "3020" ("CN") "9012" ("CN")] -> w1731
        frame "返回请求应答", Default {
        }
        frame "上传数据" {
        }
        frame "返回执行结果" {
        }
      }
      n1173 = Get Date/Time In Seconds() -> (seconds since 1Jan1904=w1729:timestamp)
      n1174 = Format Date/Time String(time format string (%c)="%Y%m%d%H%M%S%3u" ("时间格式字符串(%c)"), seconds (now)=w1729) -> (date/time string=w1728:string)  [unwired: 1 in]
      n1175 = Search and Replace String(input string=w1728, search string="." ("搜索字符串")) -> (result string=w1726:string)  [unwired: 6 in, 3 out]
    }
    frame "3092日志信息" {
      n1176 = global read "全局1.vi" "枚举"() -> (w1744:enum16{"返回请求应答", "上传数据", "返回执行结果"})
      n1177 = case shown="\"上传数据\"" w1744 {
        tunnel: ["9011" ("CN") "3092" ("CN") "9012" ("CN")] -> w1743
        frame "返回请求应答", Default {
        }
        frame "上传数据" {
        }
        frame "返回执行结果" {
        }
      }
      n1178 = Get Date/Time In Seconds() -> (seconds since 1Jan1904=w1741:timestamp)
      n1179 = Format Date/Time String(time format string (%c)="%Y%m%d%H%M%S%3u" ("时间格式字符串(%c)"), seconds (now)=w1741) -> (date/time string=w1740:string)  [unwired: 1 in]
      n1180 = Search and Replace String(input string=w1740, search string="." ("搜索字符串")) -> (result string=w1738:string)  [unwired: 6 in, 3 out]
    }
    frame "3093报警信息" {
      n1181 = global read "全局1.vi" "枚举"() -> (w1756:enum16{"返回请求应答", "上传数据", "返回执行结果"})
      n1182 = case shown="\"上传数据\"" w1756 {
        tunnel: ["9011" ("CN") "3093" ("CN") "9012" ("CN")] -> w1755
        frame "返回请求应答", Default {
        }
        frame "上传数据" {
        }
        frame "返回执行结果" {
        }
      }
      n1183 = Get Date/Time In Seconds() -> (seconds since 1Jan1904=w1753:timestamp)
      n1184 = Format Date/Time String(time format string (%c)="%Y%m%d%H%M%S%3u" ("时间格式字符串(%c)"), seconds (now)=w1753) -> (date/time string=w1752:string)  [unwired: 1 in]
      n1185 = Search and Replace String(input string=w1752, search string="." ("搜索字符串")) -> (result string=w1750:string)  [unwired: 6 in, 3 out]
    }
    frame "3090仪器参数" {
      n1186 = global read "全局1.vi" "枚举"() -> (w1768:enum16{"返回请求应答", "上传数据", "返回执行结果"})
      n1187 = case shown="\"上传数据\"" w1768 {
        tunnel: ["9011" ("CN") "3090" ("CN") "9012" ("CN")] -> w1767
        frame "返回请求应答", Default {
        }
        frame "上传数据" {
        }
        frame "返回执行结果" {
        }
      }
      n1188 = Get Date/Time In Seconds() -> (seconds since 1Jan1904=w1765:timestamp)
      n1189 = Format Date/Time String(time format string (%c)="%Y%m%d%H%M%S%3u" ("时间格式字符串(%c)"), seconds (now)=w1765) -> (date/time string=w1764:string)  [unwired: 1 in]
      n1190 = Search and Replace String(input string=w1764, search string="." ("搜索字符串")) -> (result string=w1762:string)  [unwired: 6 in, 3 out]
    }
    frame "3091校准信息" {
      n1191 = global read "全局1.vi" "枚举"() -> (w1780:enum16{"返回请求应答", "上传数据", "返回执行结果"})
      n1192 = case shown="\"上传数据\"" w1780 {
        tunnel: ["9011" ("CN") "3091" ("CN") "9012" ("CN")] -> w1779
        frame "返回请求应答", Default {
        }
        frame "上传数据" {
        }
        frame "返回执行结果" {
        }
      }
      n1193 = Get Date/Time In Seconds() -> (seconds since 1Jan1904=w1777:timestamp)
      n1194 = Format Date/Time String(time format string (%c)="%Y%m%d%H%M%S%3u" ("时间格式字符串(%c)"), seconds (now)=w1777) -> (date/time string=w1776:string)  [unwired: 1 in]
      n1195 = Search and Replace String(input string=w1776, search string="." ("搜索字符串")) -> (result string=w1774:string)  [unwired: 6 in, 3 out]
    }
    frame "提取仪器参数" {
      n1196 = global read "全局1.vi" "枚举"() -> (w1788:enum16{"返回请求应答", "上传数据", "返回执行结果"})
      n1197 = case shown="\"上传数据\"" w1788 {
        tunnel: ["9011" ("CN") "3020" ("CN") "9012" ("CN")] -> w1787
        frame "返回请求应答", Default {
        }
        frame "上传数据" {
        }
        frame "返回执行结果" {
        }
      }
      n1198 = local read "QN"() -> (w1786:string)
    }
    frame "系统状态" {
      n1199 = local read "QN"() -> (w1794:string)
    }
    frame "运行模式" {
      n1200 = local read "QN"() -> (w1798:string)
    }
    frame "测量周期" {
      n1201 = local read "QN"() -> (w1802:string)
    }
    frame "各参数测量周期" {
      n1202 = local read "QN"() -> (w1806:string)
    }
    frame "超标留样" {
      n1203 = local read "QN"() -> (w1810:string)
    }
    frame "3201告警信息" {
      n1204 = local read "QN"() -> (w1814:string)
    }
  }
  n1205 = Bundle By Name(cluster="数据块", "ST"=w26, "CN"=w29, "FLAG"=w28, "CP"=w8, "QN"=w20, "MN"="MN", "PW"="PW", "PNUM"=w6, "PNO"=w5) -> (w27:T1)
  n1206 = call "HJ212-2017.vi"("PWD？"=FALSE, "数据段"=w27) -> ("通讯包字符串"=w1:string, "通讯包"=→"通讯包":T2)  [unwired: 7 in, 1 out]
  "通讯包字符串" <- w1
  n1207 = String Length(string=w1) -> (length=→"长度":i32)
  "错误常量" <- "错误常量 2"
  "小时数据发送次数" <- 0 ("小时数据发送次数")
  "核查数据发送次数" <- 0 ("核查数据发送次数")
